vi "Parameters.vi"(8 "error in (no error)":errorcluster) -> (0 "error out":errorcluster)   [LabVIEW 2017]
uses:
  Controls/cluster.ctl
  <vilib>/addons/database/Connection.llb/Conn ObjectReference.ctl
  Controls/Plan_selection_loop.ctl
  Controls/Oven_cluster.ctl
  <vilib>/addons/database/Connection.llb/DB Tools Open Connec (Path).vi
  <vilib>/addons/database/NI_Database_API.lvlib
panel:
  out "MACHINE NAME":string[](array[string])
  out "STATION NUMBER":string[](array[string])
  out "IP Address":string[](array[string])
  in  "Home Square":bool
  in  "Tab Control":enum32{"PRESS PARAMETERS", "OVEN PARAMETERS"}(tab)
  in  "Delete Recipe":bool
  in  "Update/Create recipe":bool
  in  "Press Reciepe Name and Recipe Number":string(combo)
  in  "Press Machine":string(combo)
  in  "Press Parameters":T1 {"PRESSURE_2nd_MIN" format="%#_g bar"; "PRESSURE_1st_MIN" format="%#_g bar"; "HOLDING_TIME_MIN" format="%#_g Sec"; "MR_RETURN_TIME_MIN" format="%#_g Sec"; "PRESSURE_2nd_MAX" format="%#_g bar"; "PRESSURE_1st_MAX" format="%#_g bar"; "HOLDING_TIME_MAX" format="%#_g Sec"; "MR_RETURN_TIME_MAX" format="%#_g Sec"}
  in  "Oven Delete Recipe":bool
  in  "Oven Update/Create recipe":bool
  in  "Oven Reciepe Name and Recipe Number":string(combo)
  in  "Oven Machine":string(combo)
  in  "Oven Parameters":T2 {"Heating_time_Min" format="%#_g Sec"; "Heating_time_Max" format="%#_g Sec"; "Bottom_zone_8_Min" format="%#_g °C"; "Bottom_zone_8_Max" format="%#_g °C"; "Bottom_zone_7_Min" format="%#_g °C"; "Bottom_zone_7_Max" format="%#_g °C"; "Bottom_zone_6_Min" format="%#_g °C"; "Bottom_zone_6_Max" format="%#_g °C"; "Bottom_zone_5_Min" format="%#_g °C"; "Bottom_zone_5_Max" format="%#_g °C"; "Bottom_zone_4_Min" format="%#_g °C"; "Bottom_zone_3_Min" format="%#_g °C"; "Bottom_zone_2_Min" format="%#_g °C"; "Bottom_zone_1_Min" format="%#_g °C"; "Bottom_zone_4_Max" format="%#_g °C"; "Bottom_zone_3_Max" format="%#_g °C"; "Bottom_zone_2_Max" format="%#_g °C"; "Bottom_zone_1_Max" format="%#_g °C"; "Top_zone_8_Min" format="%#_g °C"; "Top_zone_8_Max" format="%#_g °C"; "Top_zone_7_Min" format="%#_g °C"; "Top_zone_7_Max" format="%#_g °C"; "Top_zone_6_Min" format="%#_g °C"; "Top_zone_6_Max" format="%#_g °C"; "Top_zone_5_Min" format="%#_g °C"; "Top_zone_5_Max" format="%#_g °C"; "Top_zone_4_Min" format="%#_g °C"; "Top_zone_3_Min" format="%#_g °C"; "Top_zone_2_Min" format="%#_g °C"; "Top_zone_1_Min" format="%#_g °C"; "Top_zone_4_Max" format="%#_g °C"; "Top_zone_3_Max" format="%#_g °C"; "Top_zone_2_Max" format="%#_g °C"; "Top_zone_1_Max" format="%#_g °C"}
  # "STANDARD PROCESS PARAMETERS  LOGSHEET"
  # "DAY, MONTYH, YEAR, HOURS, MINUTE, RECIPE NAME, PRODUCT COUNT"
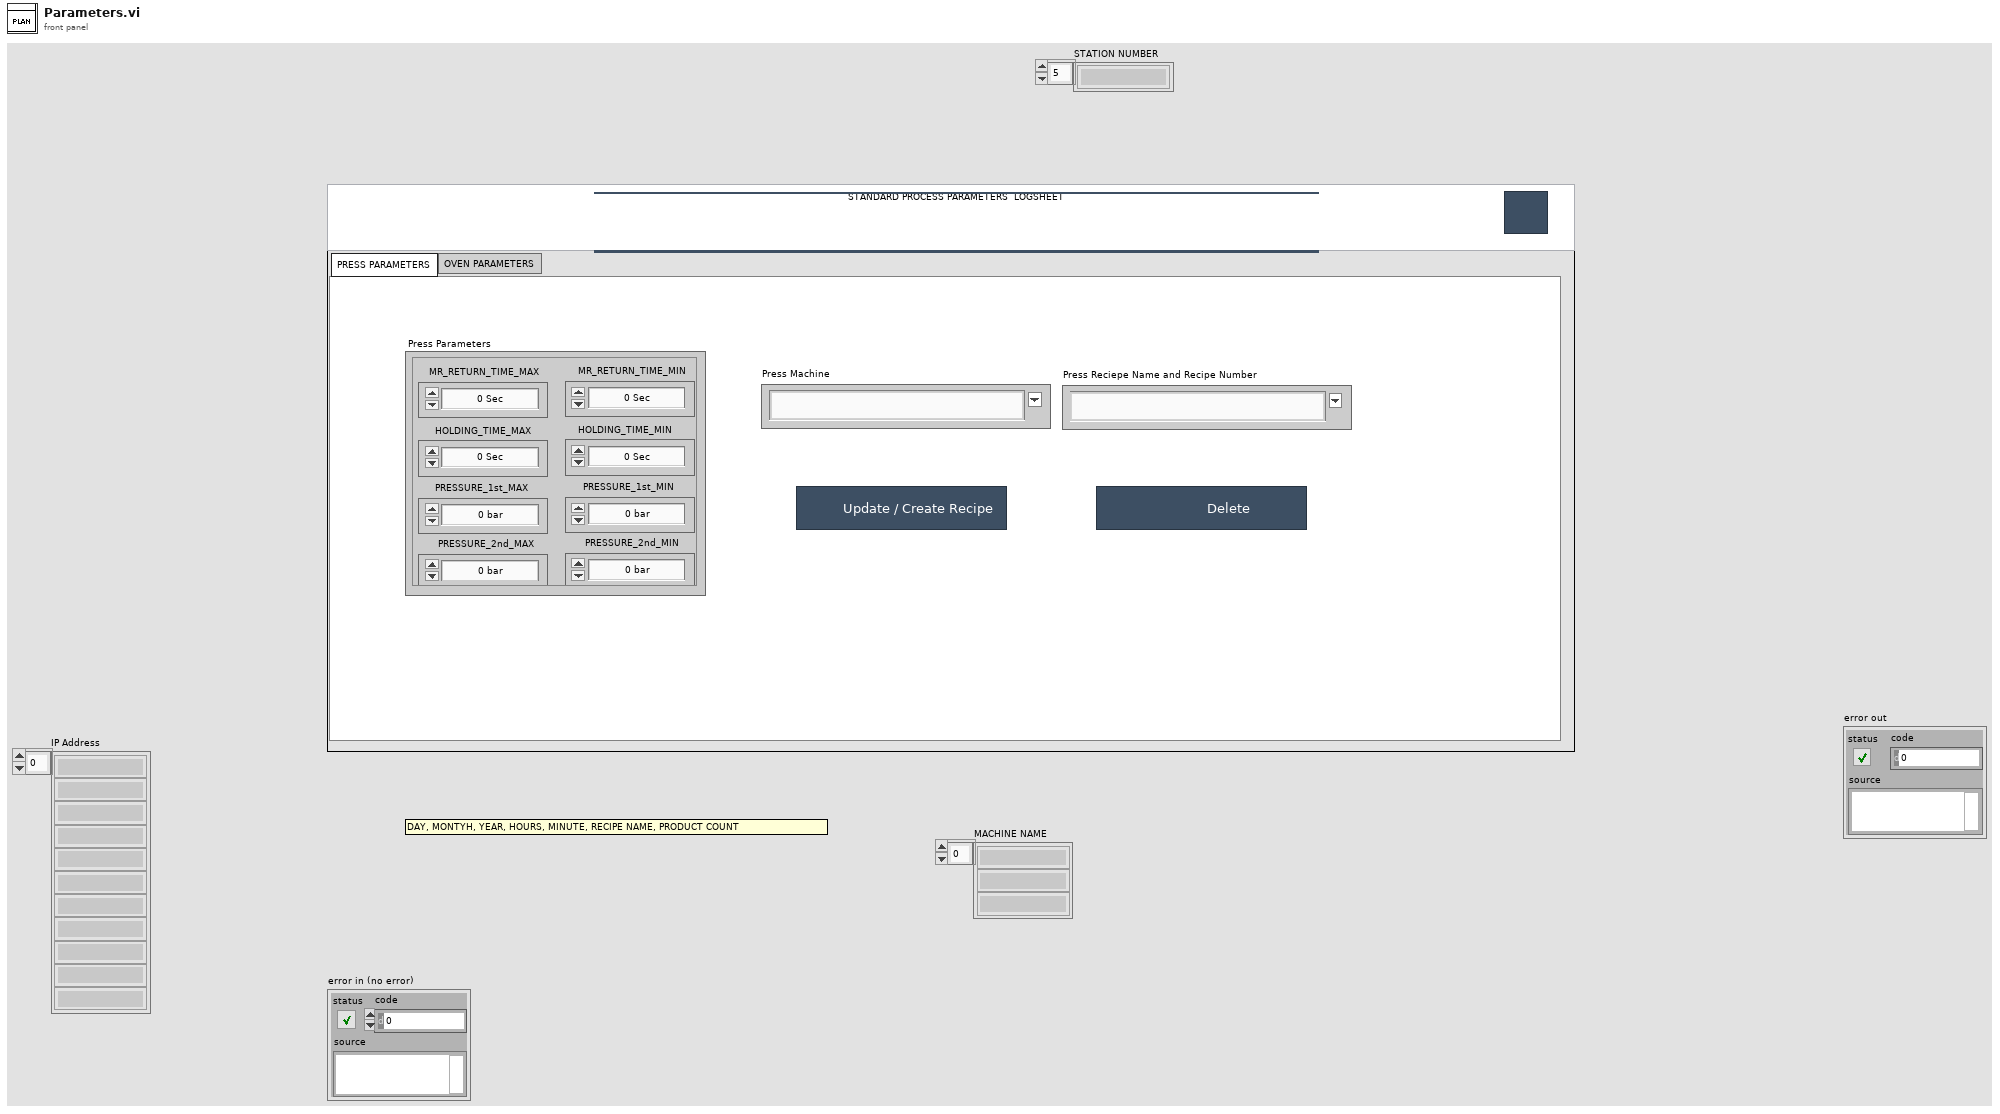
[diagram p1: front panel]
types:
  T1 = cluster{"MR_RETURN_TIME_MAX":dbl, "HOLDING_TIME_MAX":dbl, "PRESSURE_1st_MAX":dbl, "PRESSURE_2nd_MAX":dbl, "MR_RETURN_TIME_MIN":dbl, "HOLDING_TIME_MIN":dbl, "PRESSURE_1st_MIN":dbl, "PRESSURE_2nd_MIN":dbl}
  T2 = cluster{"Top_zone_1_Max":dbl, "Top_zone_1_Min":dbl, "Top_zone_2_Max":dbl, "Top_zone_2_Min":dbl, "Top_zone_3_Max":dbl, "Top_zone_3_Min":dbl, "Top_zone_4_Max":dbl, "Top_zone_4_Min":dbl, "Top_zone_5_Max":dbl, "Top_zone_5_Min":dbl, "Top_zone_6_Max":dbl, "Top_zone_6_Min":dbl, "Top_zone_7_Max":dbl, "Top_zone_7_Min":dbl, "Top_zone_8_Max":dbl, "Top_zone_8_Min":dbl, "Bottom_zone_1_Max":dbl, "Bottom_zone_1_Min":dbl, "Bottom_zone_2_Max":dbl, "Bottom_zone_2_Min":dbl, "Bottom_zone_3_Max":dbl, "Bottom_zone_3_Min":dbl, "Bottom_zone_4_Max":dbl, "Bottom_zone_4_Min":dbl, "Bottom_zone_5_Max":dbl, "Bottom_zone_5_Min":dbl, "Bottom_zone_6_Max":dbl, "Bottom_zone_6_Min":dbl, "Bottom_zone_7_Max":dbl, "Bottom_zone_7_Min":dbl, "Bottom_zone_8_Max":dbl, "Bottom_zone_8_Min":dbl, "Heating_time_Max":dbl, "Heating_time_Min":dbl}
  T3 = typedef "Oven_cluster.ctl" = cluster{"IP Address":string[], "Machine name":string[], "Station number":string[], "Product List":string[][], "Recipe_upload_history path":path, "appended array":refnum<vi>[]}
  T4 = typedef "Plan_selection_loop.ctl" = enum16{"Init", "Init_2", "Init_3", "Init_4", "Start", "Oven_Change_Recipe", "Change_Recipe", "Oven_Change_machine", "Change_machine", "Oven Save To SQL", "Save To SQL", "Oven Delete_Recipe", "Delete_Recipe", "Stop"}
  T5 = typedef "cluster.ctl" = cluster{"IP Address":string[], "Machine name":string[], "Station number":string[], "Product List":string[][], "Recipe_upload_history path":path, "reference":T6, "appended array":refnum<vi>[]}
  T6 = typedef "NI_Database_API.lvlib/Conn ObjectReference.ctl" = refnum<k1>
  T7 = cluster{"MR_RETURN_TIME_MAX":string, "HOLDING_TIME_MAX":string, "PRESSURE_1st_MAX":string, "PRESSURE_2nd_MAX":string, "MR_RETURN_TIME_MIN":string, "HOLDING_TIME_MIN":string, "PRESSURE_1st_MIN":string, "PRESSURE_2nd_MIN":string, "MACHINE_NAME":string, "RECIPE_NAME":string, "RECIPE_NUMBER":string}
  T8 = cluster{"condition[0]":dbl, "condition[1]":dbl, "condition[2]":dbl, "condition[3]":dbl, "condition[4]":dbl, "condition[5]":dbl, "condition[6]":dbl, "condition[7]":dbl}
  T9 = cluster{"condition[0]":dbl, "condition[1]":dbl, "condition[2]":dbl, "condition[3]":dbl, "condition[4]":dbl, "condition[5]":dbl, "condition[6]":dbl, "condition[7]":dbl, "condition[8]":dbl, "condition[9]":dbl, "condition[10]":dbl, "condition[11]":dbl, "condition[12]":dbl, "condition[13]":dbl, "condition[14]":dbl, "condition[15]":dbl, "condition[16]":dbl, "condition[17]":dbl, "condition[18]":dbl, "condition[19]":dbl, "condition[20]":dbl, "condition[21]":dbl, "condition[22]":dbl, "condition[23]":dbl, "condition[24]":dbl, "condition[25]":dbl, "condition[26]":dbl, "condition[27]":dbl, "condition[28]":dbl, "condition[29]":dbl, "condition[30]":dbl, "condition[31]":dbl, "condition[32]":dbl, "condition[33]":dbl}
  T10 = cluster{"Top_zone_1_Max":string, "Top_zone_2_Max":string, "Top_zone_3_Max":string, "Top_zone_4_Max":string, "Top_zone_1_Min":string, "Top_zone_2_Min":string, "Top_zone_3_Min":string, "Top_zone_4_Min":string, "Top_zone_5_Max":string, "Top_zone_5_Min":string, "Top_zone_6_Max":string, "Top_zone_6_Min":string, "Top_zone_7_Max":string, "Top_zone_7_Min":string, "Top_zone_8_Max":string, "Top_zone_8_Min":string, "Bottom_zone_1_Max":string, "Bottom_zone_2_Max":string, "Bottom_zone_3_Max":string, "Bottom_zone_4_Max":string, "Bottom_zone_1_Min":string, "Bottom_zone_2_Min":string, "Bottom_zone_3_Min":string, "Bottom_zone_4_Min":string, "Bottom_zone_5_Max":string, "Bottom_zone_5_Min":string, "Bottom_zone_6_Max":string, "Bottom_zone_6_Min":string, "Bottom_zone_7_Max":string, "Bottom_zone_7_Min":string, "Bottom_zone_8_Max":string, "Bottom_zone_8_Min":string, "Heating_time_Max":string, "Heating_time_Min":string, "MACHINE_NAME":string, "RECIPE_NAME":string, "RECIPE_NUMBER":string}
  T11 = enum32{"invalid app kind", "Development System", "Run Time System", "Student Edition", "Embedded LabVIEW", "Evaluation", "Custom"}
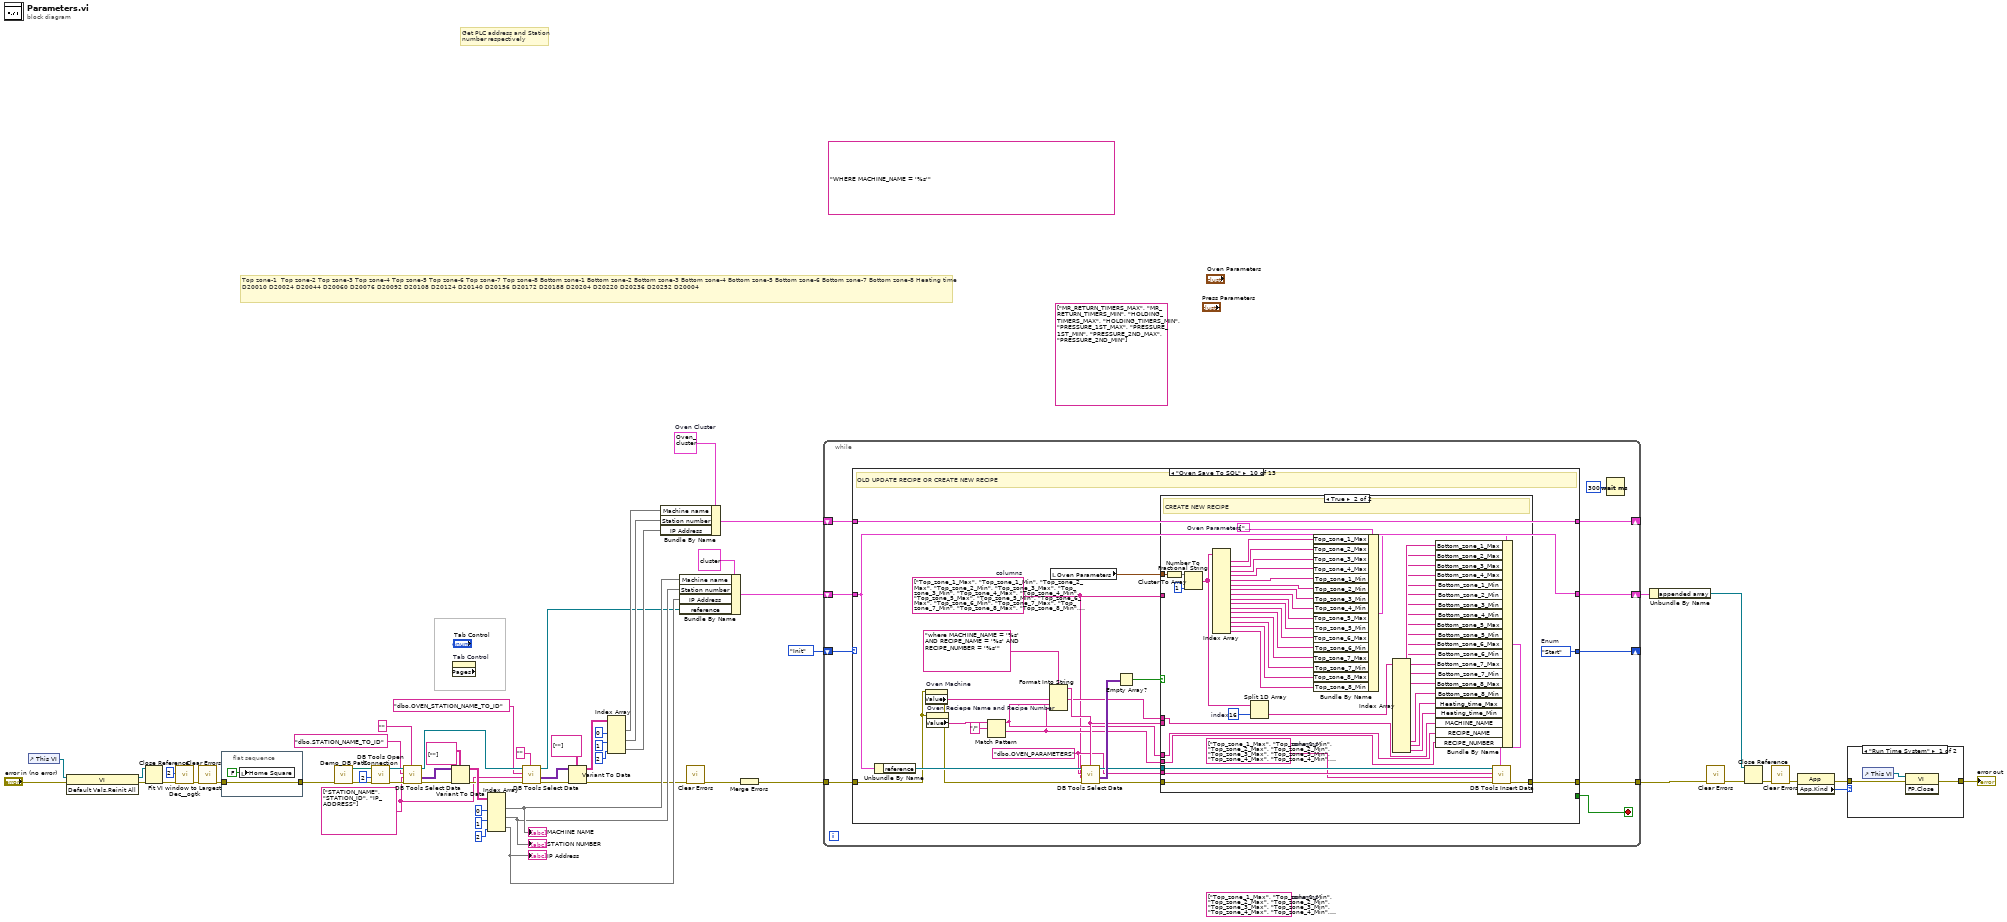
[diagram p0: block diagram]
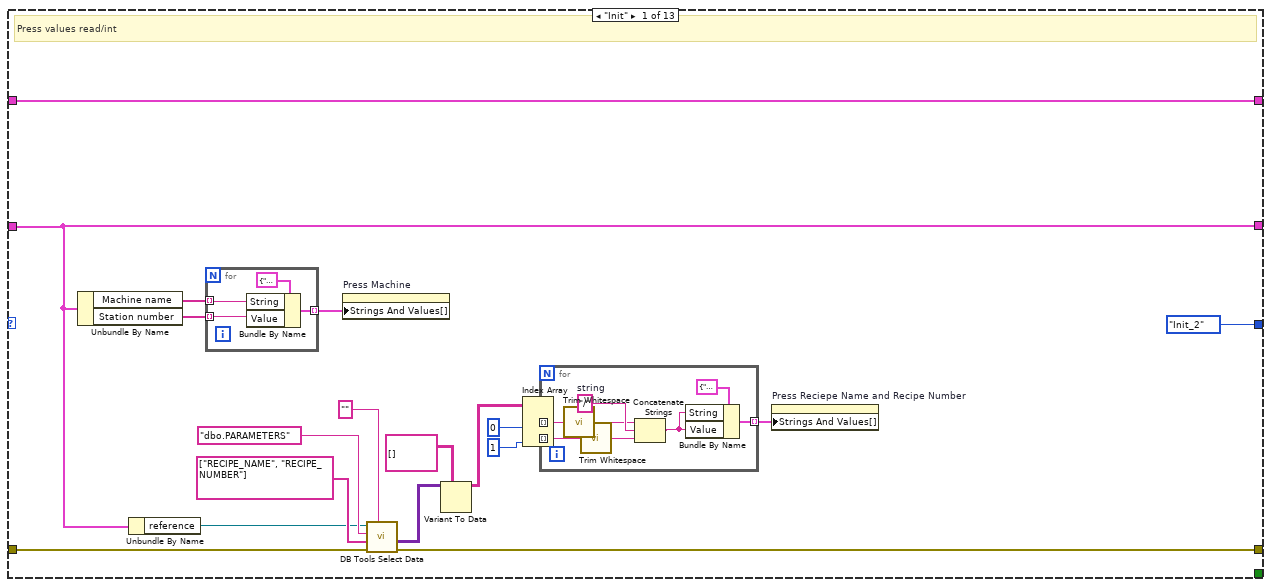
[diagram p3: hidden frame]
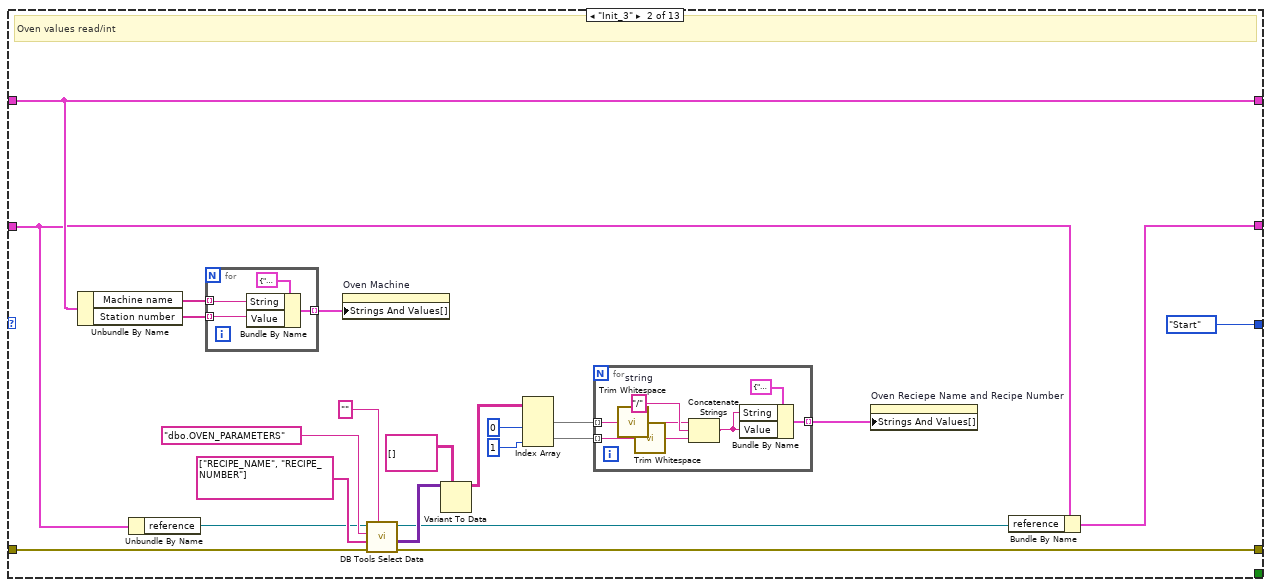
[diagram p4: hidden frame]
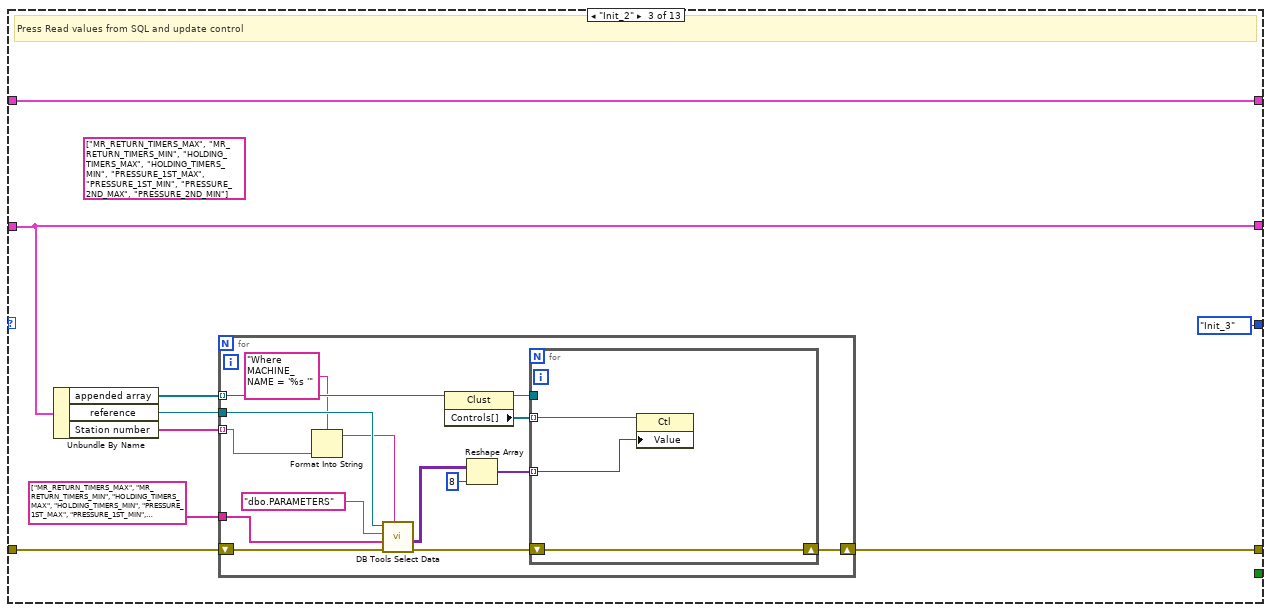
[diagram p5: hidden frame]
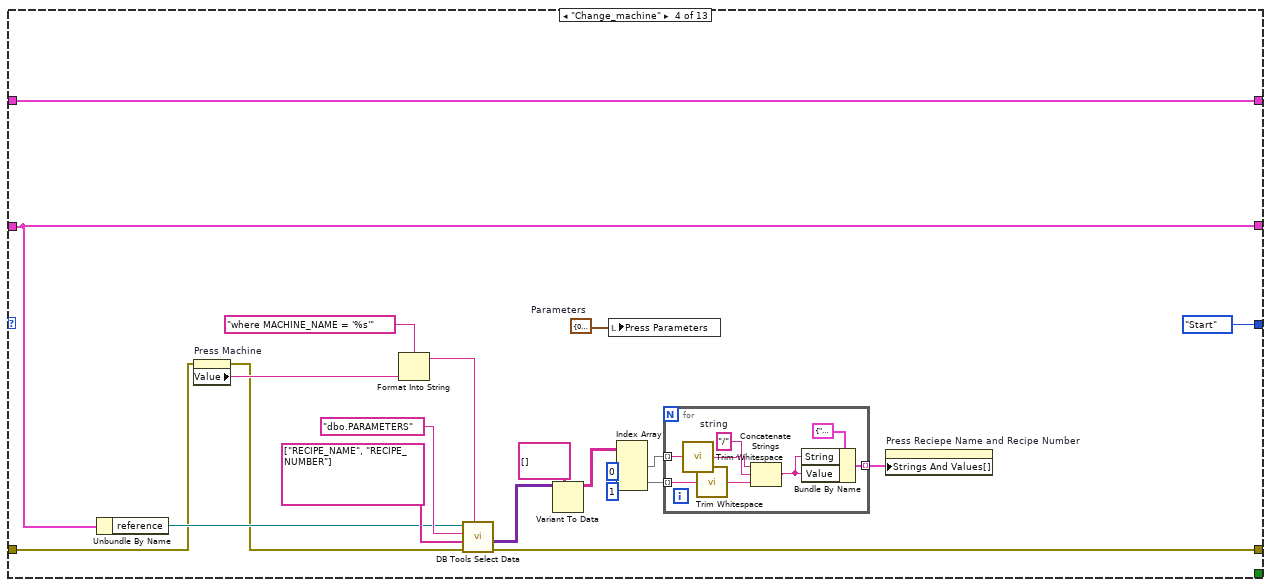
[diagram p6: hidden frame]
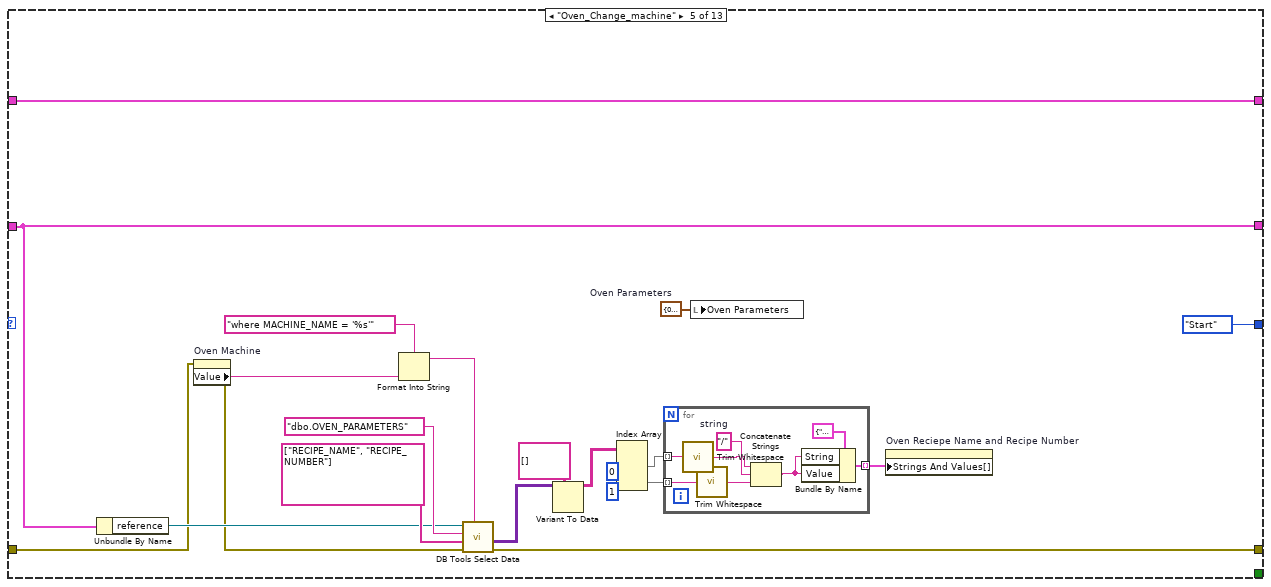
[diagram p7: hidden frame]
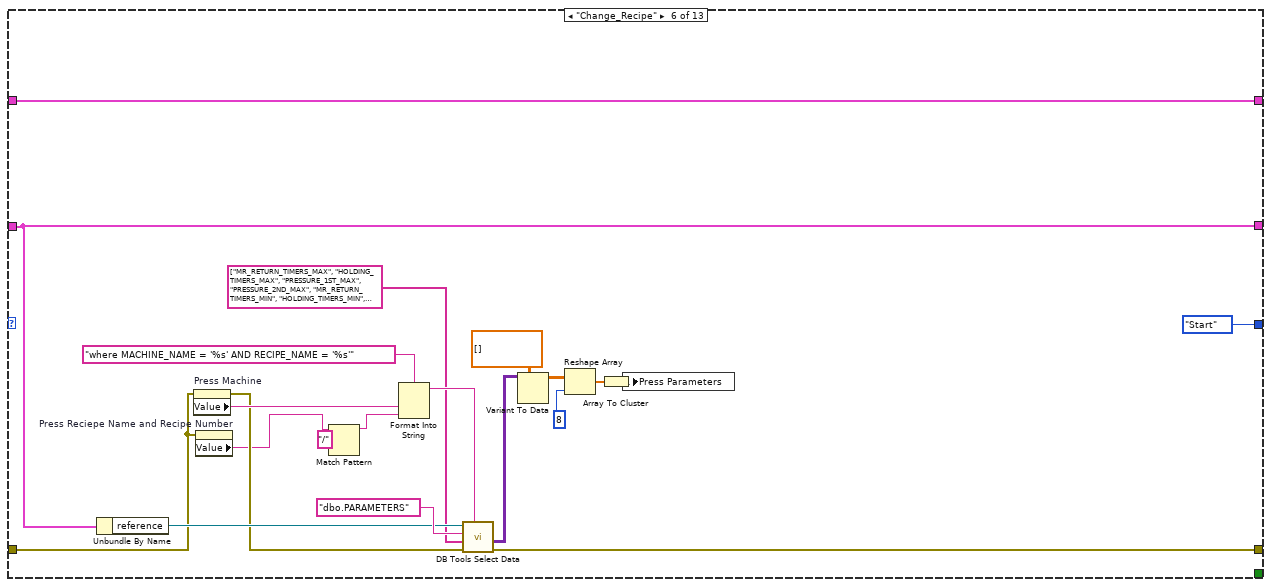
[diagram p8: hidden frame]
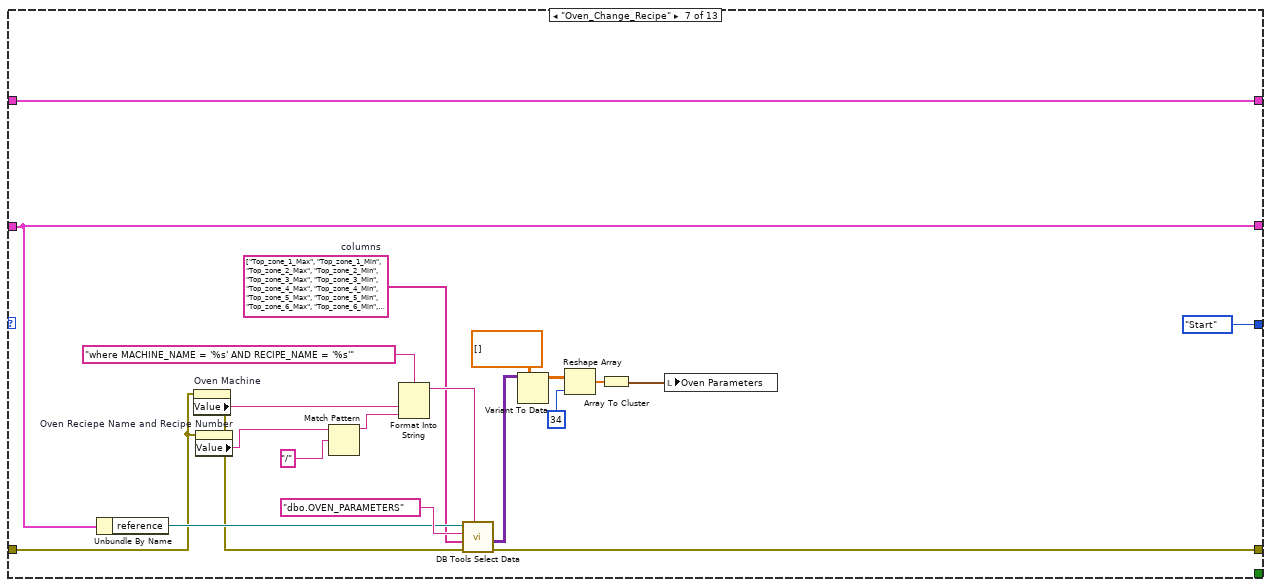
[diagram p9: hidden frame]
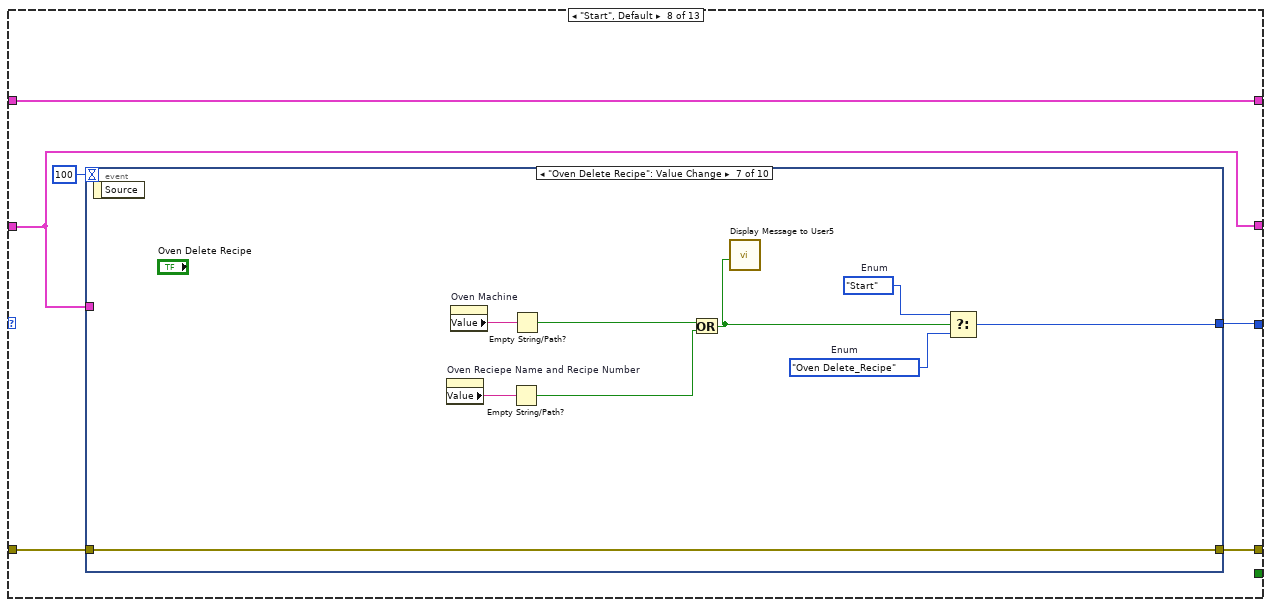
[diagram p10: hidden frame]
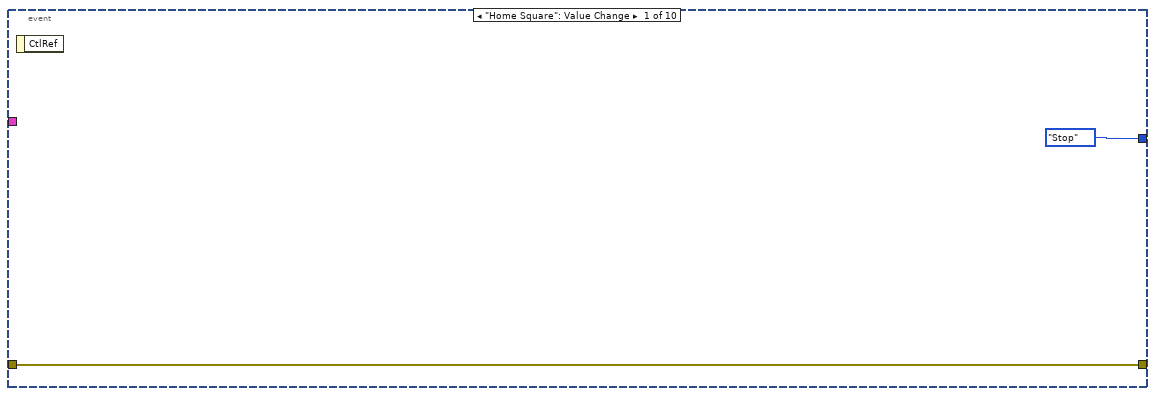
[diagram p11: hidden frame]
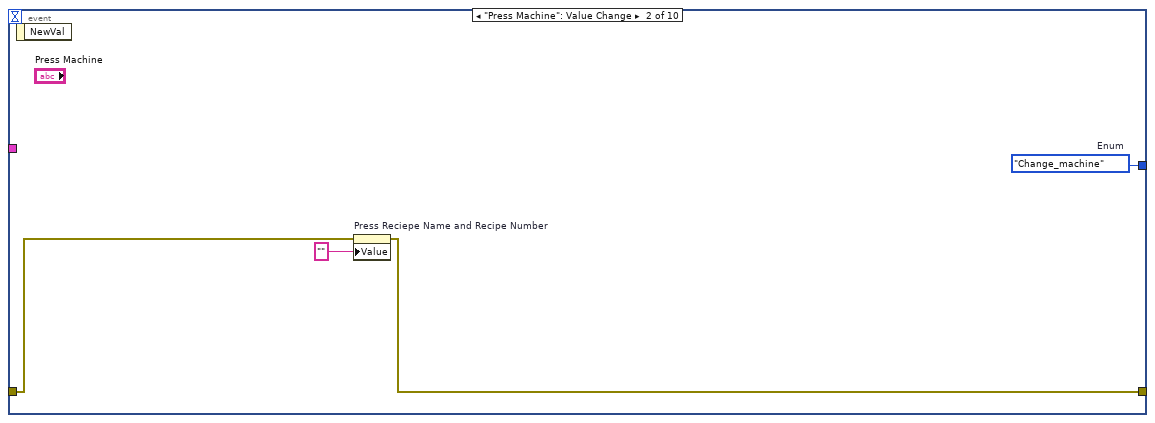
[diagram p12: hidden frame]
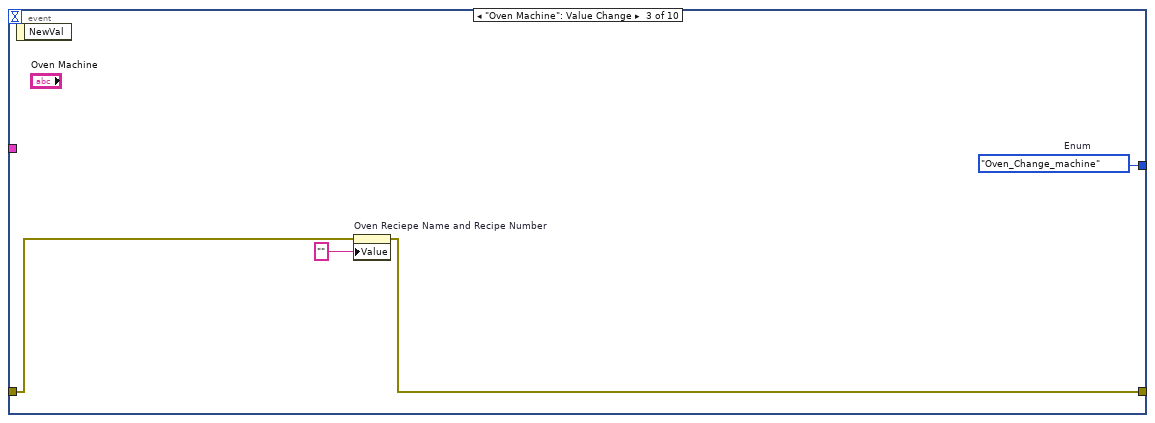
[diagram p13: hidden frame]
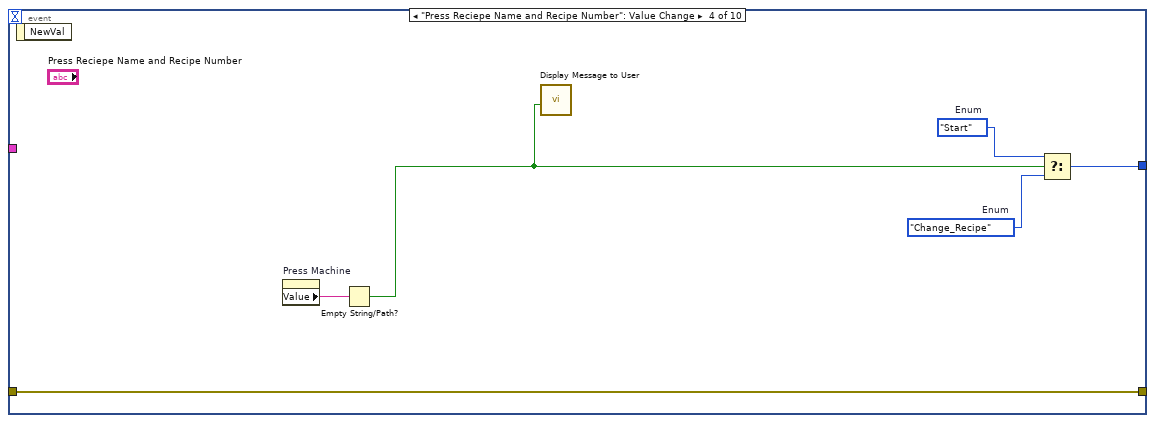
[diagram p14: hidden frame]
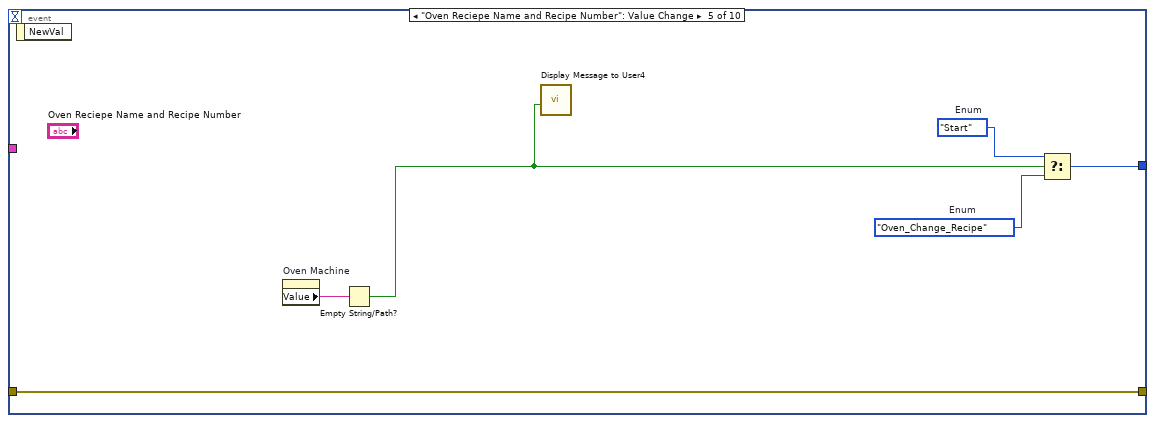
[diagram p15: hidden frame]
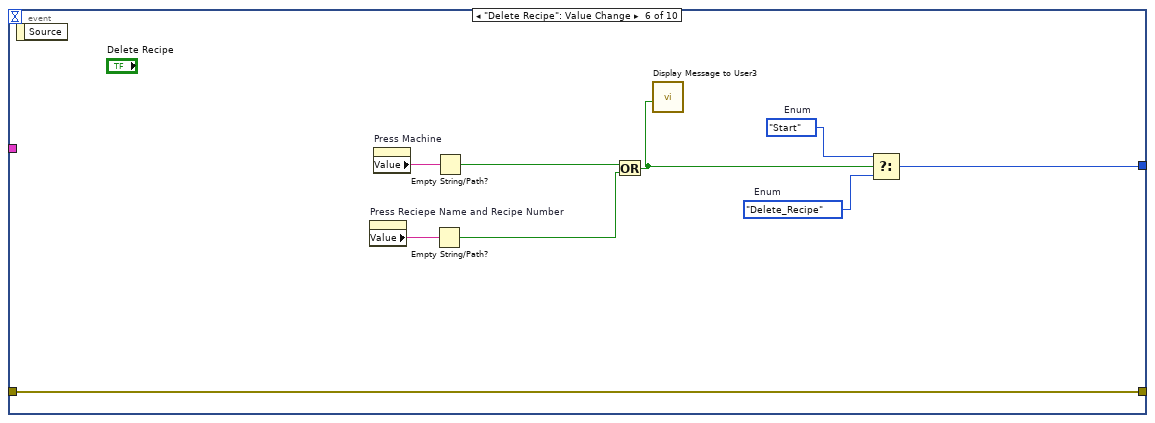
[diagram p16: hidden frame]
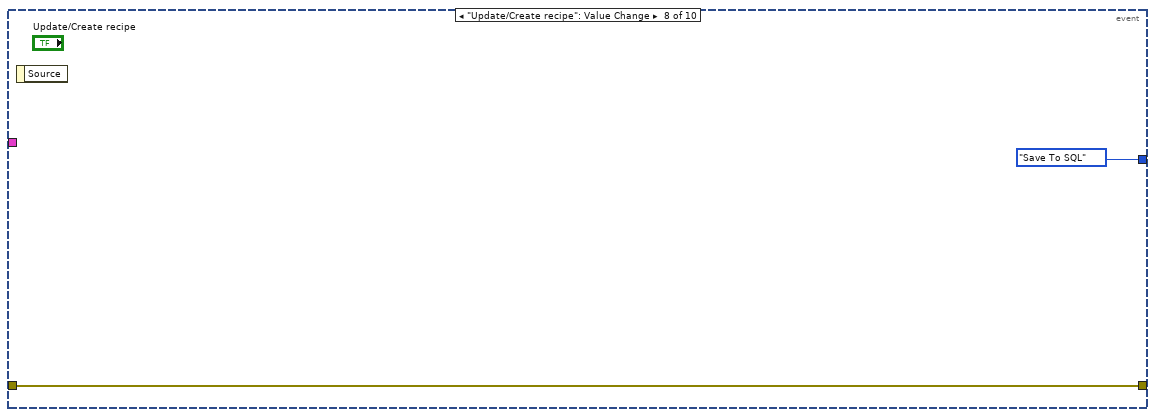
[diagram p17: hidden frame]
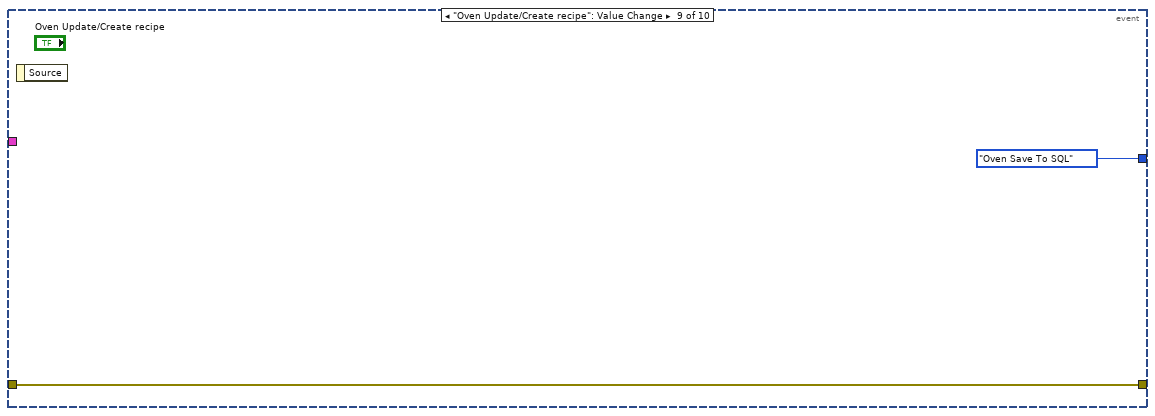
[diagram p18: hidden frame]
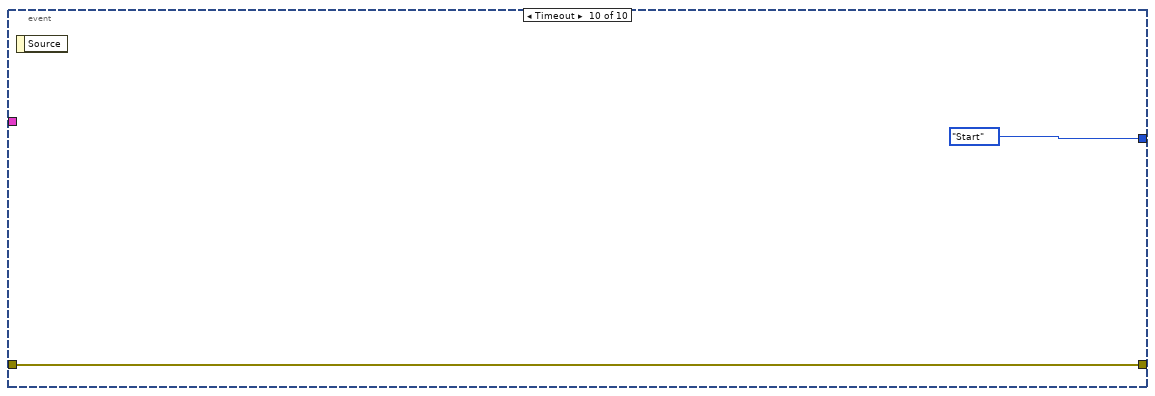
[diagram p19: hidden frame]
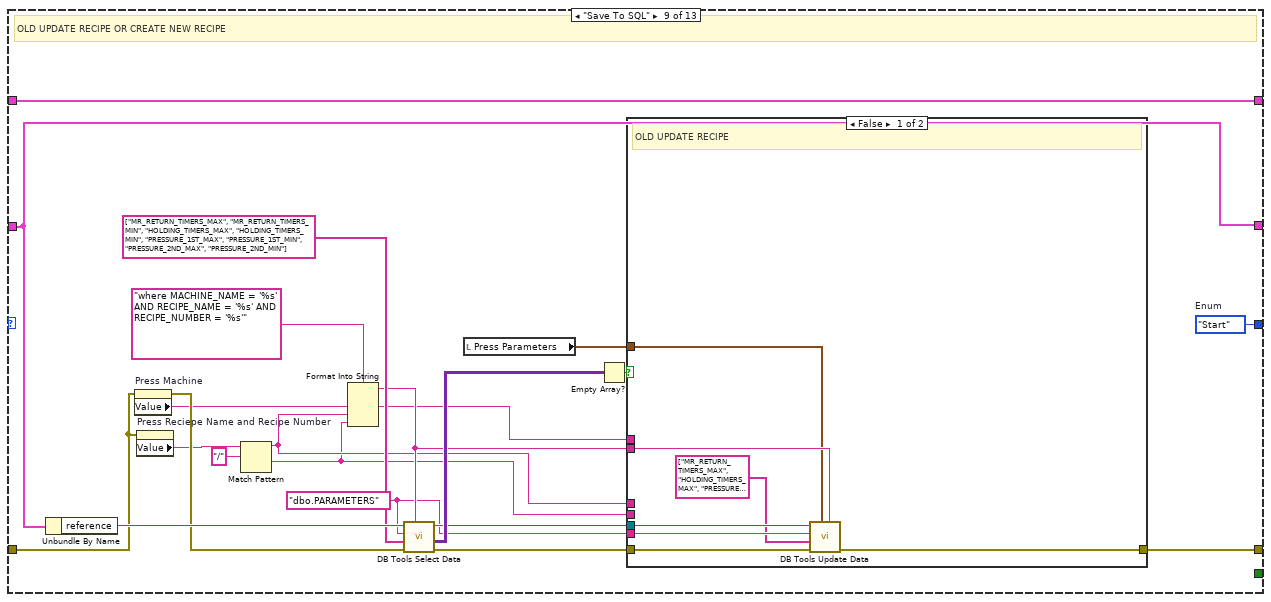
[diagram p20: hidden frame]
diagram:
  (unwired) string[] ["Top_zone_1_Max", "Top_zone_1_Min", "Top_zone_2_Max", "Top_zone_2_Min", "Top_zone_3_Max", "Top_zone_3_Min", "Top_zone_4_Max", "Top_zone_4_Min", "Top_zone_5_Max", "Top_zone_5_Min", "Top_zone_6_Max", "Top_zone_6_Min", "Top_zone_7_Max", "Top_zone_7_Min", "Top_zone_8_Max", "Top_zone_8_Min", "Bottom_zone_1_Max", "Bottom_zone_1_Min", "Bottom_zone_2_Max", "Bottom_zone_2_Min", "Bottom_zone_3_Max", "Bottom_zone_3_Min", "Bottom_zone_4_Max", "Bottom_zone_4_Min", "Bottom_zone_5_Max", "Bottom_zone_5_Min", "Bottom_zone_6_Max", "Bottom_zone_6_Min", "Bottom_zone_7_Max", "Bottom_zone_7_Min", "Bottom_zone_8_Max", "Bottom_zone_8_Min", "Heating_time_Max", "Heating_time_Min", "MACHINE_NAME", "RECIPE_NAME", "RECIPE_NUMBER"]  # columns
  w7 = T3 {"IP Address"=["", "", "", "", "", "", "", "", "", ""], "Machine name"=["", "", "", "", "", "", "", "", "", ""], "Station number"=["", "", "", "", "", "", "", "", "", ""], "Product List"=[], "Recipe_upload_history path"=path "", "appended array"=[]}  # Oven Cluster
  (unwired) string[] ["MR_RETURN_TIMERS_MAX", "MR_RETURN_TIMERS_MIN", "HOLDING_TIMERS_MAX", "HOLDING_TIMERS_MIN", "PRESSURE_1ST_MAX", "PRESSURE_1ST_MIN", "PRESSURE_2ND_MAX", "PRESSURE_2ND_MIN"] ("String")
  (unwired) "WHERE MACHINE_NAME = '%s'" ("condition")
  w17 = string[] ["STATION_NAME", "STATION_ID", "IP_ADDRESS"] ("columns")
  # "Top zone-1 \tTop zone-2\tTop zone-3\tTop zone-4\tTop zone-5\tTop zone-6\tTop zone-7\tTop zone-8\tBottom zone-1\tBottom zone-2\tBottom zone-3\tBottom zone-4\tBottom zone-5\tBottom zone-6\tBottom zone-7\tBottom zone-8\tHeating time\nD20010\tD20024\tD20044\tD20060\tD20076\tD20092\tD20108\tD20124\tD20140\tD20156\tD20172\tD20188\tD20204\tD20220\tD20236\tD20252\tD20004"
  # "Get PLC address and Station\nnumber respectively"
  n1 = control-ref of="This VI"() -> (w59:refnum<vi>)
  n2 = invoke class="VI" method="Default Vals.Reinit All"(reference=w59, error in="error in (no error)") -> (reference out=w58:refnum<vi>, error out=w57:errorcluster)  [unwired: 1 in, 1 out]
  n3 = Close Reference(reference=w58, error in (no error)=w57) -> (error out=w29:errorcluster)
  n4 = call <userlib>:"Fit VI window to Largest Dec__ogtk.vi"("error in (no error)"=w29, "border spacing (2 px)"=2) -> ("error out"=w28:errorcluster)  [unwired: 4 in, 1 out]
  n5 = call <vilib>:"Clear Errors.vi"("error in (no error)"=w28) -> ("error out"=w20:errorcluster)  [unwired: 5 in, 1 out]
  n6 = flat-sequence {
    tunnel: [w61] -> w41
    tunnel: w20 -> [w61]
    frame #0 {
      n7 = local write "Home Square"(FALSE) -> ()
    }
  }
  n8 = call "Demo_DB Path.vi"("error in"=w41) -> ("error out"=w53:errorcluster, "DB Path"=w54:path)  [unwired: 9 in]
  n9 = call-poly <vilib>:"DB Tools Open Connection.vi"("error in (no error)"=w53, "connection timeout (15)"=2, "connection information"=w54) -> ("error out"=w56:errorcluster, "connection reference"=w55:T6)  [unwired: 5 in]
  n10 = call <vilib>:"DB Tools Select Data.vi"("condition"="", "error in (no error)"=w56, "columns"=w17, "table"="dbo.STATION_NAME_TO_ID", "connection reference"=w55) -> ("error out"=w46:errorcluster, "data"=w47:variant[][], "connection reference out"=w19:T6)  [unwired: 1 in]
  n11 = Variant To Data(error in=w46, type=string[][] [[""]], Variant=w47) -> (data=w42:string[][], error out=w18:errorcluster)
  n12 = property on="Tab Control" class="TabCtl (strict)" props=["Pages"]() -> ()  [unwired: 2 in, 3 out]
  n13 = Index Array(array=w42, index (col) #1=0 ("disabled index (col)"), index (col) #2=1 ("disabled index (col)"), index (col) #3=2 ("disabled index (col)")) -> (element #1=w38:string[], element #2=w31:string[], element #3=w32:string[])  [unwired: 3 in]
  "IP Address" <- w32
  "MACHINE NAME" <- w38
  "STATION NUMBER" <- w31
  n14 = call <vilib>:"DB Tools Select Data.vi"("condition"="", "error in (no error)"=w18, "columns"=w17, "table"="dbo.OVEN_STATION_NAME_TO_ID", "connection reference"=w19) -> ("error out"=w16:errorcluster, "data"=w12:variant[][], "connection reference out"=w2:T6)  [unwired: 1 in]
  n15 = Variant To Data(error in=w16, type=string[][] [[""]], Variant=w12) -> (data=w8:string[][], error out=w15:errorcluster)
  n16 = Index Array(array=w8, index (col) #1=0 ("disabled index (col)"), index (col) #2=1 ("disabled index (col)"), index (col) #3=2 ("disabled index (col)")) -> (element #1=w5:string[], element #2=w4:string[], element #3=w3:string[])  [unwired: 3 in]
  n17 = Bundle By Name(cluster=w7, "Machine name"=w5, "Station number"=w4, "IP Address"=w3) -> (w6:T3)
  n18 = Bundle By Name(cluster=T5 {"IP Address"=["", "", "", "", "", "", "", "", "", ""], "Machine name"=["", "", "", "", "", "", "", "", "", ""], "Station number"=["", "", "", "", "", "", "", "", "", ""], "Product List"=[], "Recipe_upload_history path"=path "", "reference"=refnum, "appended array"=[]}, "Machine name"=w38, "Station number"=w31, "IP Address"=w32, "reference"=w2) -> (w40:T5)
  n19 = call <vilib>:"Clear Errors.vi"("error in (no error)"=w15) -> ("error out"=w30:errorcluster)  [unwired: 5 in, 1 out]
  n20 = Merge Errors(w30) -> (w33:errorcluster)
  n21 = while {
    tunnel: w33 -> [w70]
    shift-right: [w68] -> w35
    shift-left: w40 -> [w67]
    tunnel: [w66] -> w36
    shift-right: [w65] -> _
    shift-left: Plan_selection_loop."Init" ("Enum") -> [w69]
    shift-right: [w63] -> _
    shift-left: w6 -> [w62]
    stop <- w64 stop-if-true
    n22 = case shown="\"Oven Save To SQL\"" w69 {
      tunnel: w70 -> [w91 w125 w144 w172 w201 w233 w254 w267 w330 w381 w459 w488 w507]
      tunnel: [w81 w116 w139 w180 w209 w239 w260 w270 w318 w369 w448 w477 w506] -> w66
      tunnel: [w89 w107 w146 w184 w213 w242 w263 w266 w329 w380 w458 w487 w505] -> w68
      tunnel: w67 -> [w89 w104 w146 w184 w213 w242 w263 w266 w329 w380 w458 w487 w505]
      tunnel: [Plan_selection_loop."Init_2" ("Enum") Plan_selection_loop."Start" ("Enum") Plan_selection_loop."Init_3" ("Enum") Plan_selection_loop."Start" ("Enum") Plan_selection_loop."Start" ("Enum") Plan_selection_loop."Start" ("Enum") Plan_selection_loop."Start" ("Enum") w268 w337 w387 w447 w476 Plan_selection_loop."Stop" ("Enum")] -> w65
      tunnel: [_ _ _ _ _ _ _ _ _ _ _ _ "Home Square"] -> w64
      tunnel: [w72 w105 w138 w165 w195 w223 w245 w265 w317 w368 w446 w475 w502] -> w63
      tunnel: w62 -> [w72 w105 w138 w165 w195 w223 w245 w265 w317 w368 w446 w475 w502]
      frame "Init" {
        # "Press values read/int"
        n23 = Unbundle By Name(w89) -> ("Machine name"=w88:string[], "Station number"=w87:string[])
        n24 = Unbundle By Name(w89) -> ("reference"=w82:T6)
        n25 = for {
          tunnel: w88 -> [w102] mode=indexing
          tunnel: w87 -> [w100] mode=indexing
          tunnel: [w101] -> w86 mode=indexing
          n26 = Bundle By Name(cluster=cluster{"String":string, "Value":string} {"String"="", "Value"=""}, "String"=w102, "Value"=w100) -> (w101:cluster{"String":string, "Value":string})
        }
        n27 = property on="Press Machine" class="CmbBox"("Strings And Values[]"=w86) -> ()  [unwired: 2 in, 2 out]
        n28 = call <vilib>:"DB Tools Select Data.vi"("condition"="", "error in (no error)"=w91, "columns"=string[] ["RECIPE_NAME", "RECIPE_NUMBER"] ("String"), "table"="dbo.PARAMETERS", "connection reference"=w82) -> ("error out"=w81:errorcluster, "data"=w80:variant[][])  [unwired: 1 in, 1 out]
        n29 = Variant To Data(type=string[][] [] ("condition"), Variant=w80) -> (data=w78:string[][])  [unwired: 1 in, 1 out]
        n30 = Index Array(array=w78, index (col) #1=0, index (col) #2=1) -> (element #1=w76:string[], element #2=w73:string[])  [unwired: 2 in]
        n31 = for {
          tunnel: [w98] -> w75 mode=indexing
          tunnel: w76 -> [w94] mode=indexing
          tunnel: w73 -> [w96] mode=indexing
          w97 = "/"  # string
          n32 = call <vilib>:"Trim Whitespace.vi"("string"=w94) -> ("trimmed string"=w93:string)  [unwired: 1 in]
          n33 = call <vilib>:"Trim Whitespace.vi"("string"=w96) -> ("trimmed string"=w92:string)  [unwired: 1 in]
          n34 = Concatenate Strings(w93, w97, w92) -> (w95:string)
          n35 = Bundle By Name(cluster=cluster{"String":string, "Value":string} {"String"="", "Value"=""}, "String"=w95, "Value"=w95) -> (w98:cluster{"String":string, "Value":string})
        }
        n36 = property on="Press Reciepe Name and Recipe Number" class="CmbBox"("Strings And Values[]"=w75) -> ()  [unwired: 2 in, 2 out]
      }
      frame "Init_3" {
        # "Oven values read/int"
        n37 = Unbundle By Name(w105) -> ("Machine name"=w123:string[], "Station number"=w122:string[])
        n38 = Unbundle By Name(w104) -> ("reference"=w117:T6)
        n39 = for {
          tunnel: w123 -> [w136] mode=indexing
          tunnel: w122 -> [w134] mode=indexing
          tunnel: [w135] -> w121 mode=indexing
          n40 = Bundle By Name(cluster=cluster{"String":string, "Value":string} {"String"="", "Value"=""}, "String"=w136, "Value"=w134) -> (w135:cluster{"String":string, "Value":string})
        }
        n41 = property on="Oven Machine" class="CmbBox"("Strings And Values[]"=w121) -> ()  [unwired: 2 in, 2 out]
        n42 = call <vilib>:"DB Tools Select Data.vi"("condition"="", "error in (no error)"=w125, "columns"=string[] ["RECIPE_NAME", "RECIPE_NUMBER"] ("String"), "table"="dbo.OVEN_PARAMETERS", "connection reference"=w117) -> ("error out"=w116:errorcluster, "data"=w115:variant[][], "connection reference out"=w106:T6)  [unwired: 1 in]
        n43 = Variant To Data(type=string[][] [] ("condition"), Variant=w115) -> (data=w113:string[][])  [unwired: 1 in, 1 out]
        n44 = Index Array(array=w113, index (col) #1=0, index (col) #2=1) -> (element #1=w111:string[], element #2=w108:string[])  [unwired: 2 in]
        n45 = for {
          tunnel: [w132] -> w110 mode=indexing
          tunnel: w111 -> [w128] mode=indexing
          tunnel: w108 -> [w130] mode=indexing
          w131 = "/"  # string
          n46 = call <vilib>:"Trim Whitespace.vi"("string"=w128) -> ("trimmed string"=w127:string)  [unwired: 1 in]
          n47 = call <vilib>:"Trim Whitespace.vi"("string"=w130) -> ("trimmed string"=w126:string)  [unwired: 1 in]
          n48 = Concatenate Strings(w127, w131, w126) -> (w129:string)
          n49 = Bundle By Name(cluster=cluster{"String":string, "Value":string} {"String"="", "Value"=""}, "String"=w129, "Value"=w129) -> (w132:cluster{"String":string, "Value":string})
        }
        n50 = property on="Oven Reciepe Name and Recipe Number" class="CmbBox"("Strings And Values[]"=w110) -> ()  [unwired: 2 in, 2 out]
        n51 = Bundle By Name(cluster=w104, "reference"=w106) -> (w107:T5)
      }
      frame "Init_2" {
        (unwired) string[] ["MR_RETURN_TIMERS_MAX", "MR_RETURN_TIMERS_MIN", "HOLDING_TIMERS_MAX", "HOLDING_TIMERS_MIN", "PRESSURE_1ST_MAX", "PRESSURE_1ST_MIN", "PRESSURE_2ND_MAX", "PRESSURE_2ND_MIN"] ("String")
        # "Press Read values from SQL and update control"
        n52 = Unbundle By Name(w146) -> ("appended array"=w145:refnum<vi>[], "reference"=w140:T6, "Station number"=w142:string[])
        n53 = for {
          tunnel: w145 -> [w161] mode=indexing
          shift-right: [w160] -> w139
          shift-left: w144 -> [w157]
          tunnel: w140 -> [w154]
          tunnel: string[] ["MR_RETURN_TIMERS_MAX", "MR_RETURN_TIMERS_MIN", "HOLDING_TIMERS_MAX", "HOLDING_TIMERS_MIN", "PRESSURE_1ST_MAX", "PRESSURE_1ST_MIN", "PRESSURE_2ND_MAX", "PRESSURE_2ND_MIN"] ("String") -> [w155]
          tunnel: w142 -> [w153] mode=indexing
          n54 = Format Into String(format string="Where MACHINE_NAME = '%s '" ("condition"), w153) -> (resulting string=w150:string)  [unwired: 2 in, 1 out]
          n55 = call <vilib>:"DB Tools Select Data.vi"("condition"=w150, "error in (no error)"=w157, "columns"=w155, "table"="dbo.PARAMETERS", "connection reference"=w154) -> ("error out"=w156:errorcluster, "data"=w148:variant[][])  [unwired: 1 in, 1 out]
          n56 = property on="Property Node" class="Clust"(reference=w161) -> (reference out=w159:refnum<vi>, "Controls[]"=w158:refnum<vi>[])  [unwired: 1 in, 1 out]
          n57 = Reshape Array(w148, 8 ("dimension size")) -> (w147:variant[])
          n58 = for {
            shift-right: [w164] -> w160
            shift-left: w156 -> [w164]
            tunnel: w159 -> [_]
            tunnel: w158 -> [w163] mode=indexing
            tunnel: w147 -> [w162] mode=indexing
            n59 = property on="Property Node" class="Ctl"(reference=w163, "Value"=w162) -> ()  [unwired: 1 in, 2 out]
          }
        }
      }
      frame "Change_machine" {
        w170 = T1 {"MR_RETURN_TIME_MAX"=0.0, "HOLDING_TIME_MAX"=0.0, "PRESSURE_1st_MAX"=0.0, "PRESSURE_2nd_MAX"=0.0, "MR_RETURN_TIME_MIN"=0.0, "HOLDING_TIME_MIN"=0.0, "PRESSURE_1st_MIN"=0.0, "PRESSURE_2nd_MIN"=0.0}  # Parameters
        n60 = Unbundle By Name(w184) -> ("reference"=w181:T6)
        n61 = property on="Press Machine" class="CmbBox"(error in=w172) -> (error out=w171:errorcluster, "Value"=w175:string)  [unwired: 1 in, 1 out]
        n62 = Format Into String(format string="where MACHINE_NAME = '%s'" ("condition"), w175) -> (resulting string=w173:string)  [unwired: 2 in, 1 out]
        n63 = call <vilib>:"DB Tools Select Data.vi"("condition"=w173, "error in (no error)"=w171, "columns"=string[] ["RECIPE_NAME", "RECIPE_NUMBER"] ("String"), "table"="dbo.PARAMETERS", "connection reference"=w181) -> ("error out"=w180:errorcluster, "data"=w179:variant[][])  [unwired: 1 in, 1 out]
        n64 = Variant To Data(type=string[][] [] ("condition"), Variant=w179) -> (data=w177:string[][])  [unwired: 1 in, 1 out]
        n65 = local write "Press Parameters"(w170) -> ()
        n66 = Index Array(array=w177, index (col) #1=0, index (col) #2=1) -> (element #1=w168:string[], element #2=w166:string[])  [unwired: 2 in]
        n67 = for {
          tunnel: [w192] -> w169 mode=indexing
          tunnel: w168 -> [w188] mode=indexing
          tunnel: w166 -> [w190] mode=indexing
          w191 = "/"  # string
          n68 = call <vilib>:"Trim Whitespace.vi"("string"=w188) -> ("trimmed string"=w187:string)  [unwired: 1 in]
          n69 = call <vilib>:"Trim Whitespace.vi"("string"=w190) -> ("trimmed string"=w186:string)  [unwired: 1 in]
          n70 = Concatenate Strings(w187, w191, w186) -> (w189:string)
          n71 = Bundle By Name(cluster=cluster{"String":string, "Value":string} {"String"="", "Value"=""}, "String"=w189, "Value"=w189) -> (w192:cluster{"String":string, "Value":string})
        }
        n72 = property on="Press Reciepe Name and Recipe Number" class="CmbBox"("Strings And Values[]"=w169) -> ()  [unwired: 2 in, 2 out]
      }
      frame "Oven_Change_machine" {
        w194 = T2 {"Top_zone_1_Max"=0.0, "Top_zone_1_Min"=0.0, "Top_zone_2_Max"=0.0, "Top_zone_2_Min"=0.0, "Top_zone_3_Max"=0.0, "Top_zone_3_Min"=0.0, "Top_zone_4_Max"=0.0, "Top_zone_4_Min"=0.0, "Top_zone_5_Max"=0.0, "Top_zone_5_Min"=0.0, "Top_zone_6_Max"=0.0, "Top_zone_6_Min"=0.0, "Top_zone_7_Max"=0.0, "Top_zone_7_Min"=0.0, "Top_zone_8_Max"=0.0, "Top_zone_8_Min"=0.0, "Bottom_zone_1_Max"=0.0, "Bottom_zone_1_Min"=0.0, "Bottom_zone_2_Max"=0.0, "Bottom_zone_2_Min"=0.0, "Bottom_zone_3_Max"=0.0, "Bottom_zone_3_Min"=0.0, "Bottom_zone_4_Max"=0.0, "Bottom_zone_4_Min"=0.0, "Bottom_zone_5_Max"=0.0, "Bottom_zone_5_Min"=0.0, "Bottom_zone_6_Max"=0.0, "Bottom_zone_6_Min"=0.0, "Bottom_zone_7_Max"=0.0, "Bottom_zone_7_Min"=0.0, "Bottom_zone_8_Max"=0.0, "Bottom_zone_8_Min"=0.0, "Heating_time_Max"=0.0, "Heating_time_Min"=0.0}  # Oven Parameters
        n73 = Unbundle By Name(w213) -> ("reference"=w210:T6)
        n74 = property on="Oven Machine" class="CmbBox"(error in=w201) -> (error out=w200:errorcluster, "Value"=w204:string)  [unwired: 1 in, 1 out]
        n75 = Format Into String(format string="where MACHINE_NAME = '%s'" ("condition"), w204) -> (resulting string=w202:string)  [unwired: 2 in, 1 out]
        n76 = call <vilib>:"DB Tools Select Data.vi"("condition"=w202, "error in (no error)"=w200, "columns"=string[] ["RECIPE_NAME", "RECIPE_NUMBER"] ("String"), "table"="dbo.OVEN_PARAMETERS", "connection reference"=w210) -> ("error out"=w209:errorcluster, "data"=w208:variant[][])  [unwired: 1 in, 1 out]
        n77 = Variant To Data(type=string[][] [] ("condition"), Variant=w208) -> (data=w206:string[][])  [unwired: 1 in, 1 out]
        n78 = Index Array(array=w206, index (col) #1=0, index (col) #2=1) -> (element #1=w198:string[], element #2=w196:string[])  [unwired: 2 in]
        n79 = for {
          tunnel: [w221] -> w199 mode=indexing
          tunnel: w198 -> [w217] mode=indexing
          tunnel: w196 -> [w219] mode=indexing
          w220 = "/"  # string
          n80 = call <vilib>:"Trim Whitespace.vi"("string"=w217) -> ("trimmed string"=w216:string)  [unwired: 1 in]
          n81 = call <vilib>:"Trim Whitespace.vi"("string"=w219) -> ("trimmed string"=w215:string)  [unwired: 1 in]
          n82 = Concatenate Strings(w216, w220, w215) -> (w218:string)
          n83 = Bundle By Name(cluster=cluster{"String":string, "Value":string} {"String"="", "Value"=""}, "String"=w218, "Value"=w218) -> (w221:cluster{"String":string, "Value":string})
        }
        n84 = local write "Oven Parameters"(w194) -> ()
        n85 = property on="Oven Reciepe Name and Recipe Number" class="CmbBox"("Strings And Values[]"=w199) -> ()  [unwired: 2 in, 2 out]
      }
      frame "Change_Recipe" {
        n86 = Unbundle By Name(w242) -> ("reference"=w240:T6)
        n87 = property on="Press Machine" class="CmbBox"(error in=w233) -> (error out=w234:errorcluster, "Value"=w237:string)  [unwired: 1 in, 1 out]
        n88 = property on="Press Reciepe Name and Recipe Number" class="CmbBox"(error in=w233) -> ("Value"=w226:string)  [unwired: 1 in, 2 out]
        n89 = Match Pattern(string=w226, regular expression="/") -> (before substring=w225:string)  [unwired: 1 in, 3 out]
        n90 = Format Into String(format string="where MACHINE_NAME = '%s' AND RECIPE_NAME = '%s'" ("condition"), w237, w225) -> (resulting string=w235:string)  [unwired: 2 in, 1 out]
        n91 = call <vilib>:"DB Tools Select Data.vi"("condition"=w235, "error in (no error)"=w234, "columns"=string[] ["MR_RETURN_TIMERS_MAX", "HOLDING_TIMERS_MAX", "PRESSURE_1ST_MAX", "PRESSURE_2ND_MAX", "MR_RETURN_TIMERS_MIN", "HOLDING_TIMERS_MIN", "PRESSURE_1ST_MIN", "PRESSURE_2ND_MIN"] ("String"), "table"="dbo.PARAMETERS", "connection reference"=w240) -> ("error out"=w239:errorcluster, "data"=w230:variant[][])  [unwired: 1 in, 1 out]
        n92 = Variant To Data(type=dbl[][] [] ("condition"), Variant=w230) -> (data=w228:dbl[][])  [unwired: 1 in, 1 out]
        n93 = Reshape Array(w228, 8 ("dimension size")) -> (w231:dbl[])
        n94 = Array To Cluster(array=w231) -> (cluster=w229:T8)
        n95 = local write "Press Parameters"(w229) -> ()
      }
      frame "Oven_Change_Recipe" {
        w244 = string[] ["Top_zone_1_Max", "Top_zone_1_Min", "Top_zone_2_Max", "Top_zone_2_Min", "Top_zone_3_Max", "Top_zone_3_Min", "Top_zone_4_Max", "Top_zone_4_Min", "Top_zone_5_Max", "Top_zone_5_Min", "Top_zone_6_Max", "Top_zone_6_Min", "Top_zone_7_Max", "Top_zone_7_Min", "Top_zone_8_Max", "Top_zone_8_Min", "Bottom_zone_1_Max", "Bottom_zone_1_Min", "Bottom_zone_2_Max", "Bottom_zone_2_Min", "Bottom_zone_3_Max", "Bottom_zone_3_Min", "Bottom_zone_4_Max", "Bottom_zone_4_Min", "Bottom_zone_5_Max", "Bottom_zone_5_Min", "Bottom_zone_6_Max", "Bottom_zone_6_Min", "Bottom_zone_7_Max", "Bottom_zone_7_Min", "Bottom_zone_8_Max", "Bottom_zone_8_Min", "Heating_time_Max", "Heating_time_Min"]  # columns
        n96 = Unbundle By Name(w263) -> ("reference"=w261:T6)
        n97 = property on="Oven Machine" class="CmbBox"(error in=w254) -> (error out=w255:errorcluster, "Value"=w258:string)  [unwired: 1 in, 1 out]
        n98 = property on="Oven Reciepe Name and Recipe Number" class="CmbBox"(error in=w254) -> ("Value"=w247:string)  [unwired: 1 in, 2 out]
        n99 = Match Pattern(string=w247, regular expression="/") -> (before substring=w246:string)  [unwired: 1 in, 3 out]
        n100 = Format Into String(format string="where MACHINE_NAME = '%s' AND RECIPE_NAME = '%s'" ("condition"), w258, w246) -> (resulting string=w256:string)  [unwired: 2 in, 1 out]
        n101 = call <vilib>:"DB Tools Select Data.vi"("condition"=w256, "error in (no error)"=w255, "columns"=w244, "table"="dbo.OVEN_PARAMETERS", "connection reference"=w261) -> ("error out"=w260:errorcluster, "data"=w251:variant[][])  [unwired: 1 in, 1 out]
        n102 = Variant To Data(type=dbl[][] [] ("condition"), Variant=w251) -> (data=w249:dbl[][])  [unwired: 1 in, 1 out]
        n103 = Reshape Array(w249, 34 ("dimension size")) -> (w252:dbl[])
        n104 = Array To Cluster(array=w252) -> (cluster=w250:T9)
        n105 = local write "Oven Parameters"(w250) -> ()
      }
      frame "Start", Default {
        n106 = event shown="[6] \"Oven Delete Recipe\": Value Change" {
          selector: _ -> [_ _ _ _ _ _ _ _ _ _]
          dyn-events: _ -> [_ _ _ _ _ _ _ _ _ _]
          timeout: 100 -> [_ _ _ _ _ _ _ _ _ _]
          tunnel: [w272 w274 w278 w286 w292 w301 w310 w311 w313 w316] -> w270
          tunnel: w267 -> [w272 w276 w280 w286 w292 w301 w310 w311 w313 w316]
          tunnel: [Plan_selection_loop."Stop" ("Enum") w273 w277 w281 w287 w297 w306 Plan_selection_loop."Save To SQL" ("Enum") Plan_selection_loop."Oven Save To SQL" ("Enum") Plan_selection_loop."Start" ("Enum")] -> w268
          tunnel: w266 -> [_ _ _ _ _ _ _ _ _ _]
          event "Home Square": Value Change {
            n107 = event-data() -> ()  [unwired: 1 in, 1 out]
          }
          event "Press Machine": Value Change {
            w273 = Plan_selection_loop."Change_machine"  # Enum
            n108 = event-data() -> ()  [unwired: 1 in, 1 out]
            n109 = property on="Press Reciepe Name and Recipe Number" class="CmbBox"(error in=w276, "Value"="") -> (error out=w274:errorcluster)  [unwired: 1 in, 1 out]
          }
          event "Oven Machine": Value Change {
            w277 = Plan_selection_loop."Oven_Change_machine"  # Enum
            n110 = event-data() -> ()  [unwired: 1 in, 1 out]
            n111 = property on="Oven Reciepe Name and Recipe Number" class="CmbBox"(error in=w280, "Value"="") -> (error out=w278:errorcluster)  [unwired: 1 in, 1 out]
          }
          event "Press Reciepe Name and Recipe Number": Value Change {
            w282 = Plan_selection_loop."Start"  # Enum
            w284 = Plan_selection_loop."Change_Recipe"  # Enum
            n112 = event-data() -> ()  [unwired: 1 in, 1 out]
            n113 = property on="Press Machine" class="CmbBox"() -> ("Value"=w285:string)  [unwired: 2 in, 2 out]
            n114 = Empty String/Path?(string/path=w285) -> (empty?=w283:bool)
            n115 = call "Display Message to User"("Enable"=w283) -> ()  [unwired: 9 in, 2 out]
            n116 = Select(t=w282, s=w283, f=w284) -> (s? t:f=w281:T4)
          }
          event "Oven Reciepe Name and Recipe Number": Value Change {
            w288 = Plan_selection_loop."Start"  # Enum
            w290 = Plan_selection_loop."Oven_Change_Recipe"  # Enum
            n117 = event-data() -> ()  [unwired: 1 in, 1 out]
            n118 = property on="Oven Machine" class="CmbBox"() -> ("Value"=w291:string)  [unwired: 2 in, 2 out]
            n119 = Empty String/Path?(string/path=w291) -> (empty?=w289:bool)
            n120 = call "Display Message to User4"("Enable"=w289) -> ()  [unwired: 9 in, 2 out]
            n121 = Select(t=w288, s=w289, f=w290) -> (s? t:f=w287:T4)
          }
          event "Delete Recipe": Value Change {
            w299 = Plan_selection_loop."Start"  # Enum
            w298 = Plan_selection_loop."Delete_Recipe"  # Enum
            n122 = event-data() -> ()  [unwired: 1 in, 1 out]
            n123 = property on="Press Reciepe Name and Recipe Number" class="CmbBox"() -> ("Value"=w296:string)  [unwired: 2 in, 2 out]
            n124 = property on="Press Machine" class="CmbBox"() -> ("Value"=w300:string)  [unwired: 2 in, 2 out]
            n125 = Empty String/Path?(string/path=w296) -> (empty?=w295:bool)
            n126 = Empty String/Path?(string/path=w300) -> (empty?=w294:bool)
            n127 = Or(x=w294, y=w295) -> (x .or. y?=w293:bool)
            n128 = call "Display Message to User3"("Enable"=w293) -> ()  [unwired: 9 in, 2 out]
            n129 = Select(t=w299, s=w293, f=w298) -> (s? t:f=w297:T4)
          }
          event "Oven Delete Recipe": Value Change {
            w308 = Plan_selection_loop."Start"  # Enum
            w307 = Plan_selection_loop."Oven Delete_Recipe"  # Enum
            n130 = event-data() -> ()  [unwired: 1 in, 1 out]
            n131 = property on="Oven Reciepe Name and Recipe Number" class="CmbBox"() -> ("Value"=w305:string)  [unwired: 2 in, 2 out]
            n132 = property on="Oven Machine" class="CmbBox"() -> ("Value"=w309:string)  [unwired: 2 in, 2 out]
            n133 = Empty String/Path?(string/path=w305) -> (empty?=w304:bool)
            n134 = Empty String/Path?(string/path=w309) -> (empty?=w303:bool)
            n135 = Or(x=w303, y=w304) -> (x .or. y?=w302:bool)
            n136 = call "Display Message to User5"("Enable"=w302) -> ()  [unwired: 9 in, 2 out]
            n137 = Select(t=w308, s=w302, f=w307) -> (s? t:f=w306:T4)
          }
          event "Update/Create recipe": Value Change {
            n138 = event-data() -> ()  [unwired: 1 in, 1 out]
          }
          event "Oven Update/Create recipe": Value Change {
            n139 = event-data() -> ()  [unwired: 1 in, 1 out]
          }
          event Timeout {
            n140 = event-data() -> ()  [unwired: 1 in, 1 out]
          }
        }
      }
      frame "Save To SQL" {
        w324 = "dbo.PARAMETERS" ("table")
        w337 = Plan_selection_loop."Start"  # Enum
        # "OLD UPDATE RECIPE OR CREATE NEW RECIPE"
        n141 = Unbundle By Name(w329) -> ("reference"=w336:T6)
        n142 = property on="Press Machine" class="CmbBox"(error in=w330) -> (error out=w335:errorcluster, "Value"=w322:string)  [unwired: 1 in, 1 out]
        n143 = property on="Press Reciepe Name and Recipe Number" class="CmbBox"(error in=w330) -> ("Value"=w334:string)  [unwired: 1 in, 2 out]
        n144 = Match Pattern(string=w334, regular expression="/") -> (before substring=w321:string, after substring=w320:string)  [unwired: 1 in, 2 out]
        n145 = Format Into String(format string="where MACHINE_NAME = '%s' AND RECIPE_NAME = '%s' AND RECIPE_NUMBER = '%s'" ("condition"), w322, w321, w320) -> (resulting string=w325:string)  [unwired: 2 in, 1 out]
        n146 = call <vilib>:"DB Tools Select Data.vi"("condition"=w325, "error in (no error)"=w335, "columns"=string[] ["MR_RETURN_TIMERS_MAX", "MR_RETURN_TIMERS_MIN", "HOLDING_TIMERS_MAX", "HOLDING_TIMERS_MIN", "PRESSURE_1ST_MAX", "PRESSURE_1ST_MIN", "PRESSURE_2ND_MAX", "PRESSURE_2ND_MIN"] ("String"), "table"=w324, "connection reference"=w336) -> ("error out"=w319:errorcluster, "data"=w328:variant[][], "connection reference out"=w326:T6)  [unwired: 1 in]
        n147 = local read "Press Parameters"() -> (w323:T1)
        n148 = Empty Array?(array=w328) -> (empty?=w327:bool)
        n149 = case shown="False" w327 {
          tunnel: w319 -> [w344 w366]
          tunnel: [w343 w365] -> w318
          tunnel: w326 -> [w342 w364]
          tunnel: w325 -> [w341 _]
          tunnel: w324 -> [w340 w360]
          tunnel: w323 -> [w339 w363]
          tunnel: w322 -> [_ w350]
          tunnel: w321 -> [_ w349]
          tunnel: w320 -> [_ w348]
          frame False {
            # "OLD UPDATE RECIPE"
            n150 = call <vilib>:"DB Tools Update Data.vi"("condition"=w341, "data"=w339, "error in (no error)"=w344, "columns"=string[] ["MR_RETURN_TIMERS_MAX", "HOLDING_TIMERS_MAX", "PRESSURE_1ST_MAX", "PRESSURE_2ND_MAX", "MR_RETURN_TIMERS_MIN", "HOLDING_TIMERS_MIN", "PRESSURE_1ST_MIN", "PRESSURE_2ND_MIN"] ("String"), "table"=w340, "connection reference"=w342) -> ("error out"=w343:errorcluster)  [unwired: 4 in, 1 out]
          }
          frame True {
            # "CREATE NEW RECIPE"
            n151 = Cluster To Array(cluster=w363) -> (array=w361:dbl[])
            n152 = Number To Fractional String(number=w361, precision (6)=1) -> (F-format string=w359:string[])  [unwired: 2 in]
            n153 = Index Array(array=w359) -> (element #1=w358:string, element #2=w357:string, element #3=w356:string, element #4=w355:string, element #5=w354:string, element #6=w353:string, element #7=w352:string, element #8=w351:string)  [unwired: 8 in]
            n154 = Bundle By Name(cluster=T7 {"MR_RETURN_TIME_MAX"="", "HOLDING_TIME_MAX"="", "PRESSURE_1st_MAX"="", "PRESSURE_2nd_MAX"="", "MR_RETURN_TIME_MIN"="", "HOLDING_TIME_MIN"="", "PRESSURE_1st_MIN"="", "PRESSURE_2nd_MIN"="", "MACHINE_NAME"="", "RECIPE_NAME"="", "RECIPE_NUMBER"=""}, "MR_RETURN_TIME_MAX"=w358, "HOLDING_TIME_MAX"=w357, "PRESSURE_1st_MAX"=w356, "PRESSURE_2nd_MAX"=w355, "MR_RETURN_TIME_MIN"=w354, "HOLDING_TIME_MIN"=w353, "PRESSURE_1st_MIN"=w352, "PRESSURE_2nd_MIN"=w351, "MACHINE_NAME"=w350, "RECIPE_NAME"=w349, "RECIPE_NUMBER"=w348) -> (w347:T7)
            n155 = call <vilib>:"DB Tools Insert Data.vi"("data"=w347, "error in (no error)"=w366, "columns"=string[] ["MR_RETURN_TIMERS_MAX", "HOLDING_TIMERS_MAX", "PRESSURE_1ST_MAX", "PRESSURE_2ND_MAX", "MR_RETURN_TIMERS_MIN", "HOLDING_TIMERS_MIN", "PRESSURE_1ST_MIN", "PRESSURE_2ND_MIN", "MACHINE_NAME", "RECIPE_NAME", "RECIPE_NUMBER"] ("String"), "table"=w360, "connection reference"=w364) -> ("error out"=w365:errorcluster)  [unwired: 5 in, 1 out]
          }
        }
      }
      frame "Oven Save To SQL" {
        w367 = string[] ["Top_zone_1_Max", "Top_zone_1_Min", "Top_zone_2_Max", "Top_zone_2_Min", "Top_zone_3_Max", "Top_zone_3_Min", "Top_zone_4_Max", "Top_zone_4_Min", "Top_zone_5_Max", "Top_zone_5_Min", "Top_zone_6_Max", "Top_zone_6_Min", "Top_zone_7_Max", "Top_zone_7_Min", "Top_zone_8_Max", "Top_zone_8_Min", "Bottom_zone_1_Max", "Bottom_zone_1_Min", "Bottom_zone_2_Max", "Bottom_zone_2_Min", "Bottom_zone_3_Max", "Bottom_zone_3_Min", "Bottom_zone_4_Max", "Bottom_zone_4_Min", "Bottom_zone_5_Max", "Bottom_zone_5_Min", "Bottom_zone_6_Max", "Bottom_zone_6_Min", "Bottom_zone_7_Max", "Bottom_zone_7_Min", "Bottom_zone_8_Max", "Bottom_zone_8_Min", "Heating_time_Max", "Heating_time_Min"]  # columns
        w375 = "dbo.OVEN_PARAMETERS" ("table")
        w387 = Plan_selection_loop."Start"  # Enum
        # "OLD UPDATE RECIPE OR CREATE NEW RECIPE"
        n156 = Unbundle By Name(w380) -> ("reference"=w386:T6)
        n157 = property on="Oven Machine" class="CmbBox"(error in=w381) -> (error out=w385:errorcluster, "Value"=w373:string)  [unwired: 1 in, 1 out]
        n158 = property on="Oven Reciepe Name and Recipe Number" class="CmbBox"(error in=w381) -> ("Value"=w384:string)  [unwired: 1 in, 2 out]
        n159 = Match Pattern(string=w384, regular expression="/") -> (before substring=w372:string, after substring=w371:string)  [unwired: 1 in, 2 out]
        n160 = Format Into String(format string="where MACHINE_NAME = '%s' AND RECIPE_NAME = '%s' AND RECIPE_NUMBER = '%s'" ("condition"), w373, w372, w371) -> (resulting string=w376:string)  [unwired: 2 in, 1 out]
        n161 = local read "Oven Parameters"() -> (w374:T2)
        n162 = call <vilib>:"DB Tools Select Data.vi"("condition"=w376, "error in (no error)"=w385, "columns"=w367, "table"=w375, "connection reference"=w386) -> ("error out"=w370:errorcluster, "data"=w379:variant[][], "connection reference out"=w377:T6)  [unwired: 1 in]
        n163 = Empty Array?(array=w379) -> (empty?=w378:bool)
        n164 = case shown="True" w378 {
          tunnel: w370 -> [w394 w445]
          tunnel: [w393 w444] -> w369
          tunnel: w377 -> [w392 w443]
          tunnel: w376 -> [w391 _]
          tunnel: w375 -> [w390 w439]
          tunnel: w374 -> [w389 w442]
          tunnel: w373 -> [_ w399]
          tunnel: w372 -> [_ w398]
          tunnel: w371 -> [_ w397]
          tunnel: w367 -> [w388 _]
          frame False {
            # "OLD UPDATE RECIPE"
            n165 = call <vilib>:"DB Tools Update Data.vi"("condition"=w391, "data"=w389, "error in (no error)"=w394, "columns"=w388, "table"=w390, "connection reference"=w392) -> ("error out"=w393:errorcluster)  [unwired: 4 in, 1 out]
          }
          frame True {
            w395 = T10 {"Top_zone_1_Max"="", "Top_zone_2_Max"="", "Top_zone_3_Max"="", "Top_zone_4_Max"="", "Top_zone_1_Min"="", "Top_zone_2_Min"="", "Top_zone_3_Min"="", "Top_zone_4_Min"="", "Top_zone_5_Max"="", "Top_zone_5_Min"="", "Top_zone_6_Max"="", "Top_zone_6_Min"="", "Top_zone_7_Max"="", "Top_zone_7_Min"="", "Top_zone_8_Max"="", "Top_zone_8_Min"="", "Bottom_zone_1_Max"="", "Bottom_zone_2_Max"="", "Bottom_zone_3_Max"="", "Bottom_zone_4_Max"="", "Bottom_zone_1_Min"="", "Bottom_zone_2_Min"="", "Bottom_zone_3_Min"="", "Bottom_zone_4_Min"="", "Bottom_zone_5_Max"="", "Bottom_zone_5_Min"="", "Bottom_zone_6_Max"="", "Bottom_zone_6_Min"="", "Bottom_zone_7_Max"="", "Bottom_zone_7_Min"="", "Bottom_zone_8_Max"="", "Bottom_zone_8_Min"="", "Heating_time_Max"="", "Heating_time_Min"="", "MACHINE_NAME"="", "RECIPE_NAME"="", "RECIPE_NUMBER"=""}  # Oven Parameters
            w396 = string[] ["Top_zone_1_Max", "Top_zone_1_Min", "Top_zone_2_Max", "Top_zone_2_Min", "Top_zone_3_Max", "Top_zone_3_Min", "Top_zone_4_Max", "Top_zone_4_Min", "Top_zone_5_Max", "Top_zone_5_Min", "Top_zone_6_Max", "Top_zone_6_Min", "Top_zone_7_Max", "Top_zone_7_Min", "Top_zone_8_Max", "Top_zone_8_Min", "Bottom_zone_1_Max", "Bottom_zone_1_Min", "Bottom_zone_2_Max", "Bottom_zone_2_Min", "Bottom_zone_3_Max", "Bottom_zone_3_Min", "Bottom_zone_4_Max", "Bottom_zone_4_Min", "Bottom_zone_5_Max", "Bottom_zone_5_Min", "Bottom_zone_6_Max", "Bottom_zone_6_Min", "Bottom_zone_7_Max", "Bottom_zone_7_Min", "Bottom_zone_8_Max", "Bottom_zone_8_Min", "Heating_time_Max", "Heating_time_Min", "MACHINE_NAME", "RECIPE_NAME", "RECIPE_NUMBER"]  # columns
            w419 = 16  # index
            # "CREATE NEW RECIPE"
            n166 = Cluster To Array(cluster=w442) -> (array=w440:dbl[])
            n167 = Number To Fractional String(number=w440, precision (6)=1) -> (F-format string=w420:string[])  [unwired: 2 in]
            n168 = Index Array(array=w420) -> (element #1=w438:string, element #2=w437:string, element #3=w436:string, element #4=w435:string, element #5=w434:string, element #6=w433:string, element #7=w432:string, element #8=w431:string, element #9=w430:string, element #10=w429:string, element #11=w428:string, element #12=w427:string, element #13=w426:string, element #14=w425:string, element #15=w424:string, element #16=w423:string)  [unwired: 16 in]
            n169 = Split 1D Array(array=w420, index=w419) -> (second subarray=w418:string[])  [unwired: 1 out]
            n170 = Bundle By Name(cluster=w395, "Top_zone_1_Max"=w438, "Top_zone_2_Max"=w437, "Top_zone_3_Max"=w436, "Top_zone_4_Max"=w435, "Top_zone_1_Min"=w434, "Top_zone_2_Min"=w433, "Top_zone_3_Min"=w432, "Top_zone_4_Min"=w431, "Top_zone_5_Max"=w430, "Top_zone_5_Min"=w429, "Top_zone_6_Max"=w428, "Top_zone_6_Min"=w427, "Top_zone_7_Max"=w426, "Top_zone_7_Min"=w425, "Top_zone_8_Max"=w424, "Top_zone_8_Min"=w423) -> (w422:T10)
            n171 = Index Array(array=w418) -> (element #1=w417:string, element #2=w416:string, element #3=w415:string, element #4=w414:string, element #5=w413:string, element #6=w412:string, element #7=w411:string, element #8=w410:string, element #9=w409:string, element #10=w408:string, element #11=w407:string, element #12=w406:string, element #13=w405:string, element #14=w404:string, element #15=w403:string, element #16=w402:string, element #17=w401:string, element #18=w400:string)  [unwired: 18 in]
            n172 = Bundle By Name(cluster=w422, "Bottom_zone_1_Max"=w417, "Bottom_zone_2_Max"=w416, "Bottom_zone_3_Max"=w415, "Bottom_zone_4_Max"=w414, "Bottom_zone_1_Min"=w413, "Bottom_zone_2_Min"=w412, "Bottom_zone_3_Min"=w411, "Bottom_zone_4_Min"=w410, "Bottom_zone_5_Max"=w409, "Bottom_zone_5_Min"=w408, "Bottom_zone_6_Max"=w407, "Bottom_zone_6_Min"=w406, "Bottom_zone_7_Max"=w405, "Bottom_zone_7_Min"=w404, "Bottom_zone_8_Max"=w403, "Bottom_zone_8_Min"=w402, "Heating_time_Max"=w401, "Heating_time_Min"=w400, "MACHINE_NAME"=w399, "RECIPE_NAME"=w398, "RECIPE_NUMBER"=w397) -> (w421:T10)
            n173 = call <vilib>:"DB Tools Insert Data.vi"("data"=w421, "error in (no error)"=w445, "columns"=w396, "table"=w439, "connection reference"=w443) -> ("error out"=w444:errorcluster)  [unwired: 5 in, 1 out]
          }
        }
      }
      frame "Delete_Recipe" {
        w453 = "dbo.PARAMETERS" ("table")
        # "Delete Selected Recipe"
        n174 = Unbundle By Name(w458) -> ("reference"=w465:T6)
        n175 = property on="Press Machine" class="CmbBox"(error in=w459) -> (error out=w464:errorcluster, "Value"=w452:string)  [unwired: 1 in, 1 out]
        n176 = property on="Press Reciepe Name and Recipe Number" class="CmbBox"(error in=w459) -> ("Value"=w463:string)  [unwired: 1 in, 2 out]
        n177 = Match Pattern(string=w463, regular expression="/") -> (before substring=w451:string, after substring=w450:string)  [unwired: 1 in, 2 out]
        n178 = Format Into String(format string="where MACHINE_NAME = '%s' AND RECIPE_NAME = '%s' AND RECIPE_NUMBER = '%s'" ("condition"), w452, w451, w450) -> (resulting string=w454:string)  [unwired: 2 in, 1 out]
        n179 = call <vilib>:"DB Tools Select Data.vi"("condition"=w454, "error in (no error)"=w464, "columns"=string[] ["MR_RETURN_TIMERS_MAX", "MR_RETURN_TIMERS_MIN", "HOLDING_TIMERS_MAX", "HOLDING_TIMERS_MIN", "PRESSURE_1ST_MAX", "PRESSURE_1ST_MIN", "PRESSURE_2ND_MAX", "PRESSURE_2ND_MIN"] ("String"), "table"=w453, "connection reference"=w465) -> ("error out"=w449:errorcluster, "data"=w457:variant[][], "connection reference out"=w455:T6)  [unwired: 1 in]
        n180 = Empty Array?(array=w457) -> (empty?=w456:bool)
        n181 = case shown="False" w456 {
          tunnel: w449 -> [w471 w473]
          tunnel: [w470 w473] -> w448
          tunnel: w455 -> [w469 _]
          tunnel: w454 -> [w468 _]
          tunnel: w453 -> [w467 _]
          tunnel: w452 -> [_ _]
          tunnel: w451 -> [_ _]
          tunnel: w450 -> [_ _]
          tunnel: [w466 w472] -> w447
          frame False {
            w466 = Plan_selection_loop."Change_Recipe"  # Enum
            # "Delete Recipe"
            n182 = call <vilib>:"DB Tools Delete Data.vi"("condition"=w468, "error in (no error)"=w471, "table"=w467, "connection reference"=w469) -> ("error out"=w470:errorcluster)  [unwired: 6 in, 1 out]
          }
          frame True {
            w472 = Plan_selection_loop."Start"  # Enum
            # "No recipe Present"
            n183 = call "Display Message to User2"() -> ()  [unwired: 10 in, 2 out]
          }
        }
      }
      frame "Oven Delete_Recipe" {
        w474 = string[] ["Top_zone_1_Max", "Top_zone_1_Min", "Top_zone_2_Max", "Top_zone_2_Min", "Top_zone_3_Max", "Top_zone_3_Min", "Top_zone_4_Max", "Top_zone_4_Min", "Top_zone_5_Max", "Top_zone_5_Min", "Top_zone_6_Max", "Top_zone_6_Min", "Top_zone_7_Max", "Top_zone_7_Min", "Top_zone_8_Max", "Top_zone_8_Min", "Bottom_zone_1_Max", "Bottom_zone_1_Min", "Bottom_zone_2_Max", "Bottom_zone_2_Min", "Bottom_zone_3_Max", "Bottom_zone_3_Min", "Bottom_zone_4_Max", "Bottom_zone_4_Min", "Bottom_zone_5_Max", "Bottom_zone_5_Min", "Bottom_zone_6_Max", "Bottom_zone_6_Min", "Bottom_zone_7_Max", "Bottom_zone_7_Min", "Bottom_zone_8_Max", "Bottom_zone_8_Min", "Heating_time_Max", "Heating_time_Min"]  # columns
        w482 = "dbo.OVEN_PARAMETERS" ("table")
        # "Oven Delete Selected Recipe"
        n184 = Unbundle By Name(w487) -> ("reference"=w493:T6)
        n185 = property on="Oven Machine" class="CmbBox"(error in=w488) -> (error out=w492:errorcluster, "Value"=w481:string)  [unwired: 1 in, 1 out]
        n186 = property on="Oven Reciepe Name and Recipe Number" class="CmbBox"(error in=w488) -> ("Value"=w491:string)  [unwired: 1 in, 2 out]
        n187 = Match Pattern(string=w491, regular expression="/") -> (before substring=w480:string, after substring=w479:string)  [unwired: 1 in, 2 out]
        n188 = Format Into String(format string="where MACHINE_NAME = '%s' AND RECIPE_NAME = '%s' AND RECIPE_NUMBER = '%s'" ("condition"), w481, w480, w479) -> (resulting string=w483:string)  [unwired: 2 in, 1 out]
        n189 = call <vilib>:"DB Tools Select Data.vi"("condition"=w483, "error in (no error)"=w492, "columns"=w474, "table"=w482, "connection reference"=w493) -> ("error out"=w478:errorcluster, "data"=w486:variant[][], "connection reference out"=w484:T6)  [unwired: 1 in]
        n190 = Empty Array?(array=w486) -> (empty?=w485:bool)
        n191 = case shown="False" w485 {
          tunnel: w478 -> [w499 w501]
          tunnel: [w498 w501] -> w477
          tunnel: w484 -> [w497 _]
          tunnel: w483 -> [w496 _]
          tunnel: w482 -> [w495 _]
          tunnel: w481 -> [_ _]
          tunnel: w480 -> [_ _]
          tunnel: w479 -> [_ _]
          tunnel: [w494 w500] -> w476
          frame False {
            w494 = Plan_selection_loop."Oven_Change_Recipe"  # Enum
            # "Delete Recipe"
            n192 = call <vilib>:"DB Tools Delete Data.vi"("condition"=w496, "error in (no error)"=w499, "table"=w495, "connection reference"=w497) -> ("error out"=w498:errorcluster)  [unwired: 6 in, 1 out]
          }
          frame True {
            w500 = Plan_selection_loop."Start"  # Enum
            # "No recipe Present"
            n193 = call "Display Message to User6"() -> ()  [unwired: 10 in, 2 out]
          }
        }
      }
      frame "Stop" {
        n194 = Unbundle By Name(w505) -> ("reference"=w504:T6)
        n195 = call <vilib>:"DB Tools Close Connection.vi"("error in (no error)"=w507, "connection reference"=w504) -> ("error out"=w506:errorcluster)  [unwired: 5 in]
      }
    }
    n196 = Wait (ms)(milliseconds to wait=u32 300) -> ()  [unwired: 1 out]
  }
  n197 = Unbundle By Name(w35) -> ("appended array"=w34:refnum<vi>[])
  n198 = call <vilib>:"Clear Errors.vi"("error in (no error)"=w36) -> ("error out"=w37:errorcluster)  [unwired: 5 in, 1 out]
  n199 = Close Reference(reference=w34, error in (no error)=w37) -> (error out=w23:errorcluster)
  n200 = call <vilib>:"Clear Errors.vi"("error in (no error)"=w23) -> ("error out"=w24:errorcluster)  [unwired: 5 in, 1 out]
  n201 = property class="App"(error in=w24) -> (error out=w26:errorcluster, "App.Kind"=w25:T11)  [unwired: 1 in, 1 out]
  n202 = case shown="\"Run Time System\"" w25 {
    tunnel: [w509 w512] -> w22
    tunnel: w26 -> [w510 w512]
    frame "Run Time System" {
      n203 = control-ref of="This VI"() -> (w511:refnum<vi>)
      n204 = invoke class="VI" method="FP.Close"(reference=w511, error in=w510) -> (error out=w509:errorcluster)  [unwired: 1 in, 2 out]
    }
    frame "Development System", Default {
    }
  }
  "error out" <- w22
